vi "Query_Dust_Event_v2.vi"(8 "error in (no error)":errorcluster) -> (0 "error out":errorcluster)   [LabVIEW 2015]
uses:
  Controls/Constraints.ctl
  Controls/Graph.ctl
  Controls/Waveforms.ctl
  <vilib>/Utility/miscctls.llb/LVPointTypeDef.ctl
  <vilib>/addons/h5labview/H5F_mode.ctl
  <userlib>/_OpenG.lib/array/array.llb/Remove Duplicates from 1D Array (String)__ogtk.vi
  <userlib>/_OpenG.lib/array/array.llb/Empty 1D Array (Variant)__ogtk.vi
  <userlib>/_OpenG.lib/array/array.llb/Search 1D Array (String)__ogtk.vi
  <userlib>/_OpenG.lib/array/array.llb/Empty 1D Array (I32)__ogtk.vi
  <userlib>/_OpenG.lib/array/array.llb/Index 1D Array Elements (String)__ogtk.vi
  <userlib>/_OpenG.lib/array/array.llb/Search 1D Array (I32)__ogtk.vi
  <userlib>/_OpenG.lib/array/array.llb/Delete Elements from 1D Array (I32)__ogtk.vi
  <userlib>/_OpenG.lib/array/array.llb/Search 1D Array (Variant)__ogtk.vi
  <userlib>/_OpenG.lib/comparison/comparison.llb/Boolean Changed__ogtk.vi
  <vilib>/Utility/file.llb/Write To Spreadsheet File (string).vi
  <userlib>/_OpenG.lib/array/array.llb/Search 1D Array (U64)__ogtk.vi
  <userlib>/_OpenG.lib/array/array.llb/Sort 1D Array (U64)__ogtk.vi
  <userlib>/_OpenG.lib/array/array.llb/Delete Elements from 1D Array (U64)__ogtk.vi
  <vilib>/addons/h5labview/H5File.lvlib
panel:
  out "Updating...":bool
  out "Week":dbl
  out "Last Metadata Name":string
  in  "Tab Control":T1(tab)
  in  "Limit to":i64=10000 min=0 step=1000
  in  "Limit no. of\nplotted events":bool=TRUE
  in  "Experiment Group":string
  in  "Plot":bool
  in  "Select Names":bool
  in  "Save Plot Metadata":bool caption="Save Metadata"
  in  "Show Names":bool
  out "Plotted Metadata Slide":u8(slide) scale=0.0..100.0
  in  "Save Image":bool
  out "Plot Radius?":bool
  out "Constrained Distribution":T2
  in  "Experiment Name":string
  in  "Save Plot Waveforms":bool caption="Save Waveforms"
  out "Plotted Waveforms Slide":u8(slide) scale=0.0..100.0
  in  "Reset Constraints to Default":bool
  out "Number of Matching Events:":i32
  out "Description for Experiment Name:":string caption="Experiment Description:"
  out "Percentage of triggers that fit constraints:":dbl format="%#_4g%"
  out "Total Number of triggers:":i64
  in  "Constraints":T3={"Upper Timestamp Range"=timestamp(0 s since 1904-01-01), "Lower Timestamp Range"=timestamp(0 s since 1904-01-01), "Experiment Group:"="", "Experiment Name:"=[], "Upper Velocity Limit (km/s)"=299792.0, "Lower Velocity Limit (km/s)"=0.0, "Upper Mass Limit (kg)"=1.0, "Lower Mass Limit (kg)"=0.0, "name array"=[], "Estimate Quality"={0.0, 5.0}} {"Estimate Quality" scale=-5.0..5.0; "Lower Mass Limit (kg)" min=-1.0 max=1.0 step=1e-20; "Upper Mass Limit (kg)" min=-1.0 max=1.0 step=1e-20; "Lower Velocity Limit (km/s)" min=-1.0 max=299792000.0; "Upper Velocity Limit (km/s)" min=-1.0 max=299792000.0}
  out "Dust Type":string
  in  "Radius (µm)":dbl=2.0
  in  "Mass (kg)":dbl=2.638602750087072e-13 min=1e-20 max=1e-10
  in  "Velocity (km/s)":dbl=1.0 min=0.001 max=200.0
  out "Density (g/cc)":dbl
  in  "Reset Visible Time":bool caption="Save Metadata"
  out "Number of selected waveforms":i32=10
  in  "Select None":bool
  in  "Select All":bool
  in  "Selected?":bool
  in  "Limit waveforms to":i64=10
  in  "Plot Waveforms":bool
  in  "Show errored waveforms":bool
  in  "Set to plot constraints":bool
  out "Waveforms":T4[](array[typedef])
  in  "Waveform Select Names":bool
  in  "Waveforms Experiment Name":string
  in  "Waveform Show Names":bool
  in  "Waveforms Experiment Group":string
  in  "Waveform Constraints":T3 {"Estimate Quality" scale=0.0..5.0; "Lower Mass Limit (kg)" min=0.0 step=1e-20; "Upper Mass Limit (kg)" min=0.0 step=1e-20}
  out "Selected Waveforms":u64[](array[numeric])
  out "Selected Waveforms Slide":u8(slide) scale=0.0..100.0
  in  "Save Selected Waveforms":bool caption="Save Waveforms"
  out "Selected Metadata Slide":u8(slide) scale=0.0..100.0
  in  "Save Selected Metadata":bool caption="Save Metadata"
  in  "Time Visible":dbl=5000.0 min=0.0 step=1000.0
  out "Max Time":dbl=5000.0
  out "Multipliers":dbl[](array[numeric])
  in  "If this was the big acc...":bool
  in  "Sensitivity:":dbl=12100000000000.0
  in  "Vnoise Estimate:":dbl=0.005
  in  "Pelletron Voltage (MV):":dbl=2.17 caption="Needle Voltage (MV):"
  out "Test":bool caption="Test Database in use:"
  out "Test 2":bool caption="Production Database in use:"
  in  "Small?":bool
  in  "Clear Errors":bool
  in  "Exit":bool
  # "Query Dust Event V2"
  # "Go to Desktop/Accelerator/Documentation/SQL Column Translations.xlsx\nfor info about the Estimate Quality metric"
  # "events"
  # "Cursor"
  # "events"
  # "Plot Settings:"
  # "Error Status:"
  # "ODBC Connection Status:"
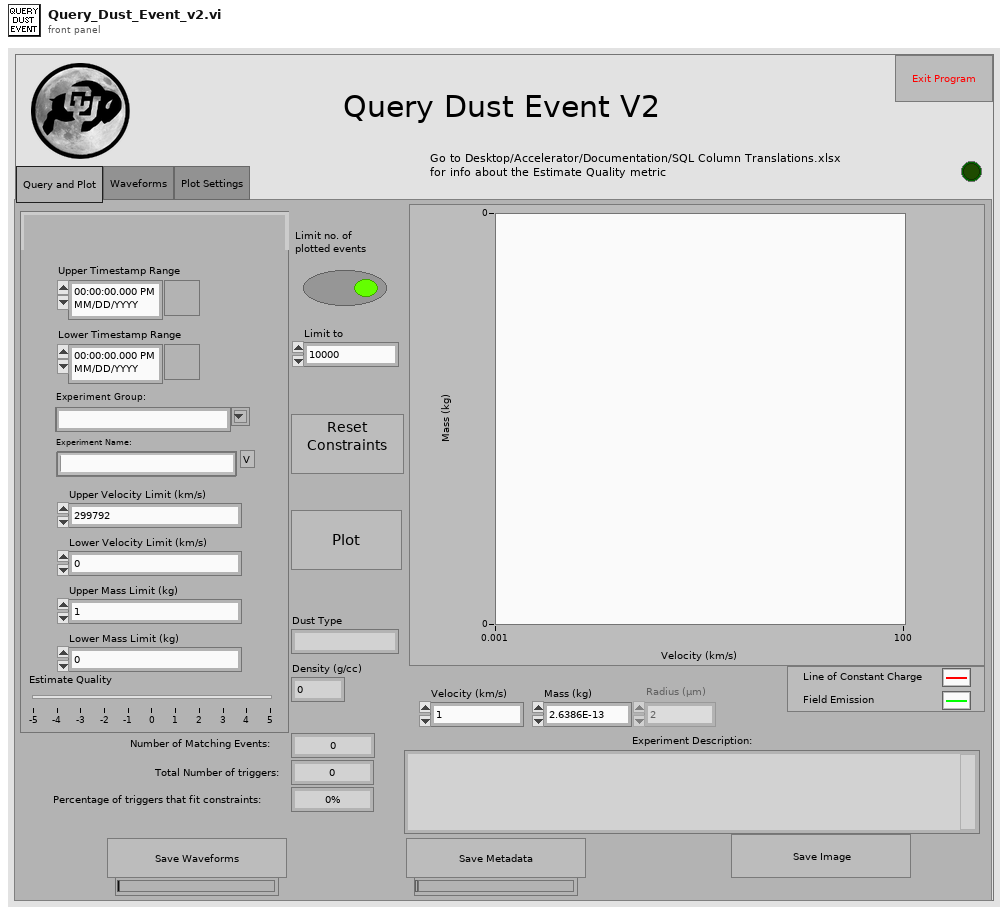
[diagram p1: front panel]
types:
  T1 = enum32{"Query and Plot", "Waveforms", "Plot Settings"}
  T2 = typedef "Graph.ctl" = cluster{cluster{"Vnoise":dbl, "Vnoise":dbl}[]}[]
  T3 = typedef "Constraints.ctl" = cluster{"Upper Timestamp Range":timestamp, "Lower Timestamp Range":timestamp, "Experiment Group:":string, "Experiment Name:":i32[], "Upper Velocity Limit (km/s)":dbl, "Lower Velocity Limit (km/s)":dbl, "Upper Mass Limit (kg)":dbl, "Lower Mass Limit (kg)":dbl, "name array":string[], "Estimate Quality":cluster{dbl, dbl}}
  T4 = typedef "Waveforms.ctl" = cluster{"id_dust_event":u64, "Time Stamp":timestamp, "Velocity":dbl, "Mass":dbl, "Charge":dbl, "Radius":dbl, "Waveform Graph":sgl[][], "Quality":i32}
  T5 = enum8{"Enabled", "Disabled", "Disabled and Grayed Out"}
  T6 = typedef "LVPointTypeDef.ctl" = cluster{"Horizontal":i16, "Vertical":i16}
  T7 = typedef "H5File.lvlib/H5F_mode.ctl" = enum16{"read-only", "read-write", "overwrite", "create new", "open or create"}
  T8 = typedef "Query_Dust_Event.ctl" = cluster{"Dust Event ID":i64, "Integer Timestamp":i64, "Velocity":dbl, "Mass":dbl, "Charge":sgl, "Radius":sgl, "Passed_3rd_Detector":i8, "High Voltage":sgl, "+ High Voltage Supply":sgl, "- High Voltage Supply":sgl, "HV Control Difference":sgl, "Vacuum Pressure":sgl, "Radiation":sgl, "Column Current":sgl, "Lost Charge":sgl, "Chain Current":sgl, "Control High Voltage":sgl, "Current Group Name:":string, "Current Experiment Name:":string, "Current Experiment Description:":string, "Estimate Source":T9, "Estimate Quality":i8, "File Location":T10, "Dust Type":string, "Dust Density":sgl}
  T9 = typedef "Estimate_source.ctl" = i8
  T10 = typedef "File_location.ctl" = i8
  T11 = cluster{"Upper Timestamp Range":timestamp, "Lower Timestamp Range":timestamp, "Experiment Group:":string, "Experiment Name:":i32[], "Upper Velocity Limit (km/s)":dbl, "Lower Velocity Limit (km/s)":dbl, "Upper Mass Limit (kg)":dbl, "Lower Mass Limit (kg)":dbl, "name array":string[], "Estimate Quality":cluster{dbl, dbl}}
  T12 = typedef "imagedata.ctl" = cluster{"image type":i32, "image depth":i32, "image":u8[], "mask":u8[], "colors":u32[], "Rectangle":cluster{"left":i16, "top":i16, "right":i16, "bottom":i16}}
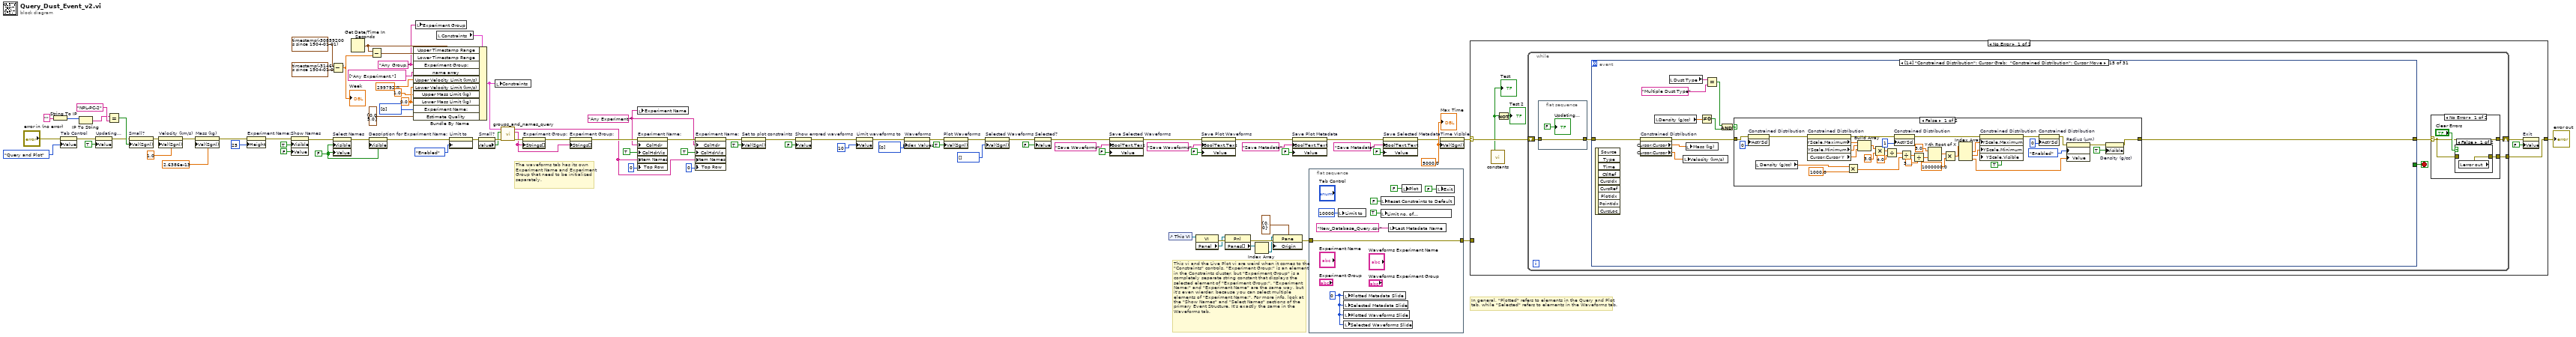
[diagram p0: block diagram]
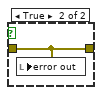
[diagram p2: hidden frame]
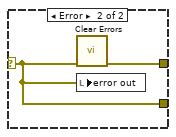
[diagram p3: hidden frame]
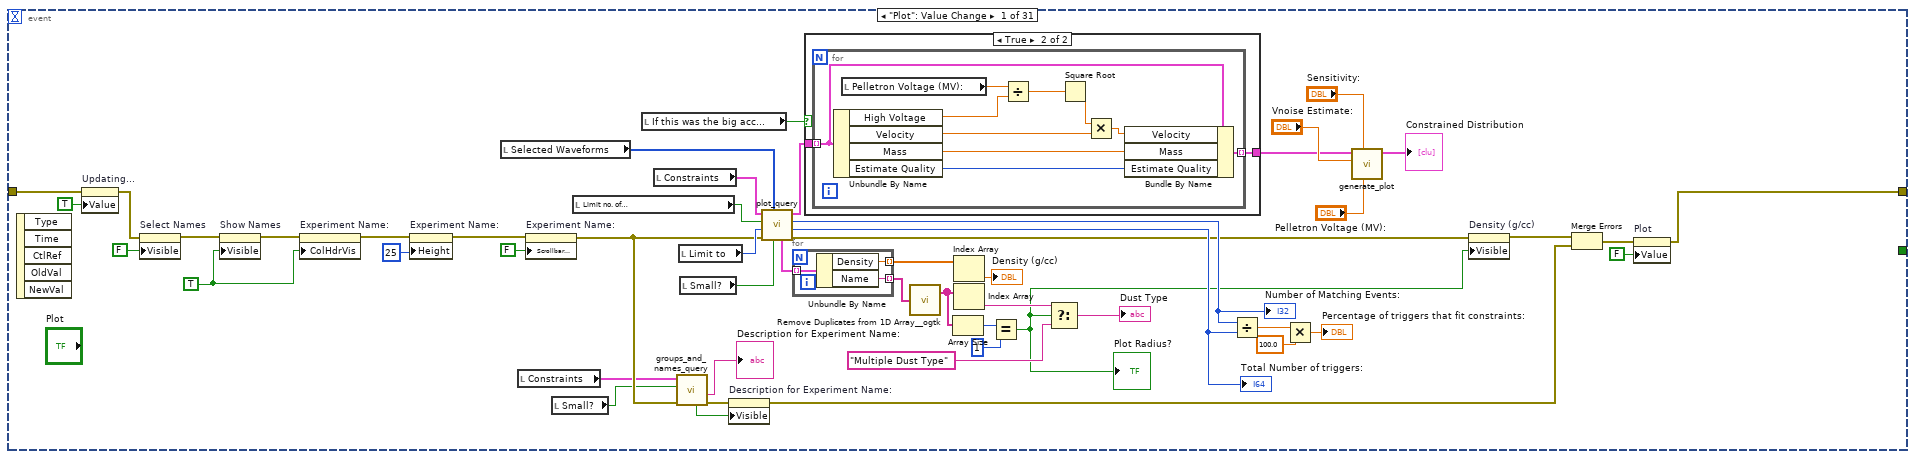
[diagram p4: hidden frame]
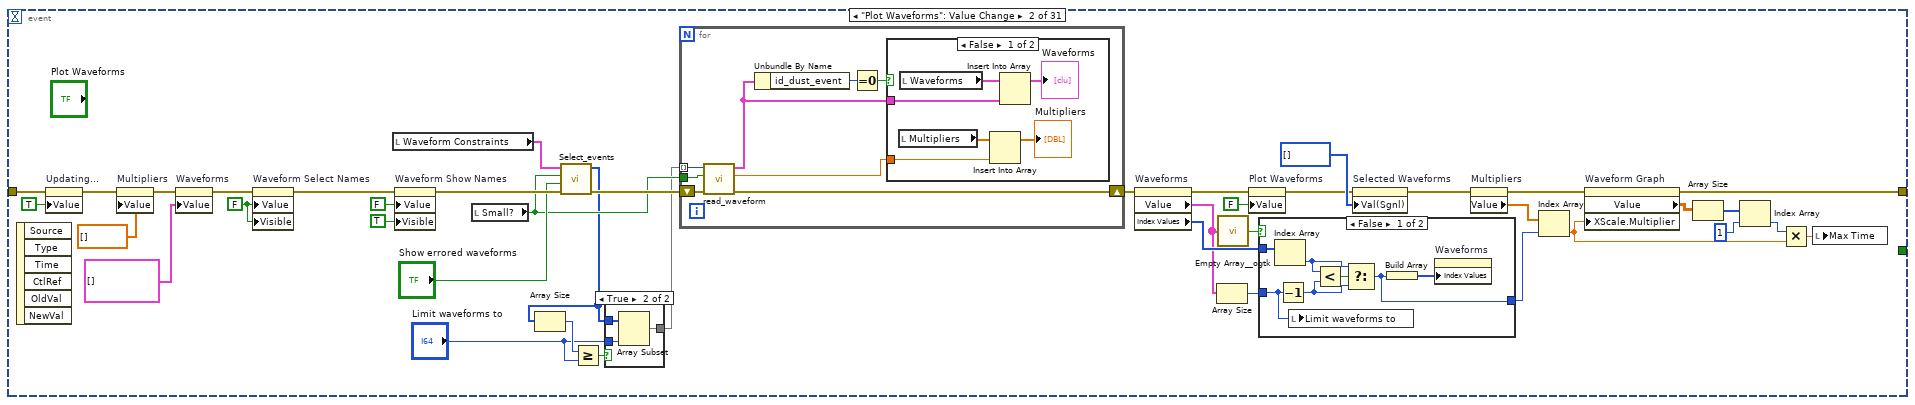
[diagram p6: hidden frame]
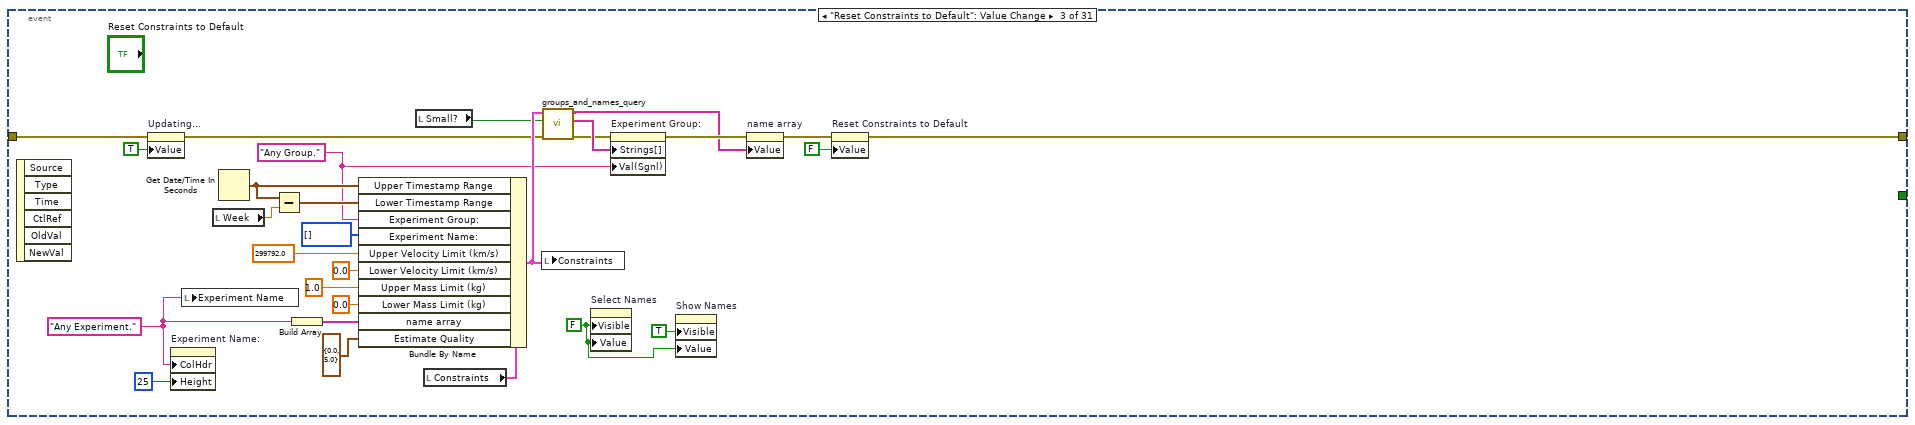
[diagram p10: hidden frame]
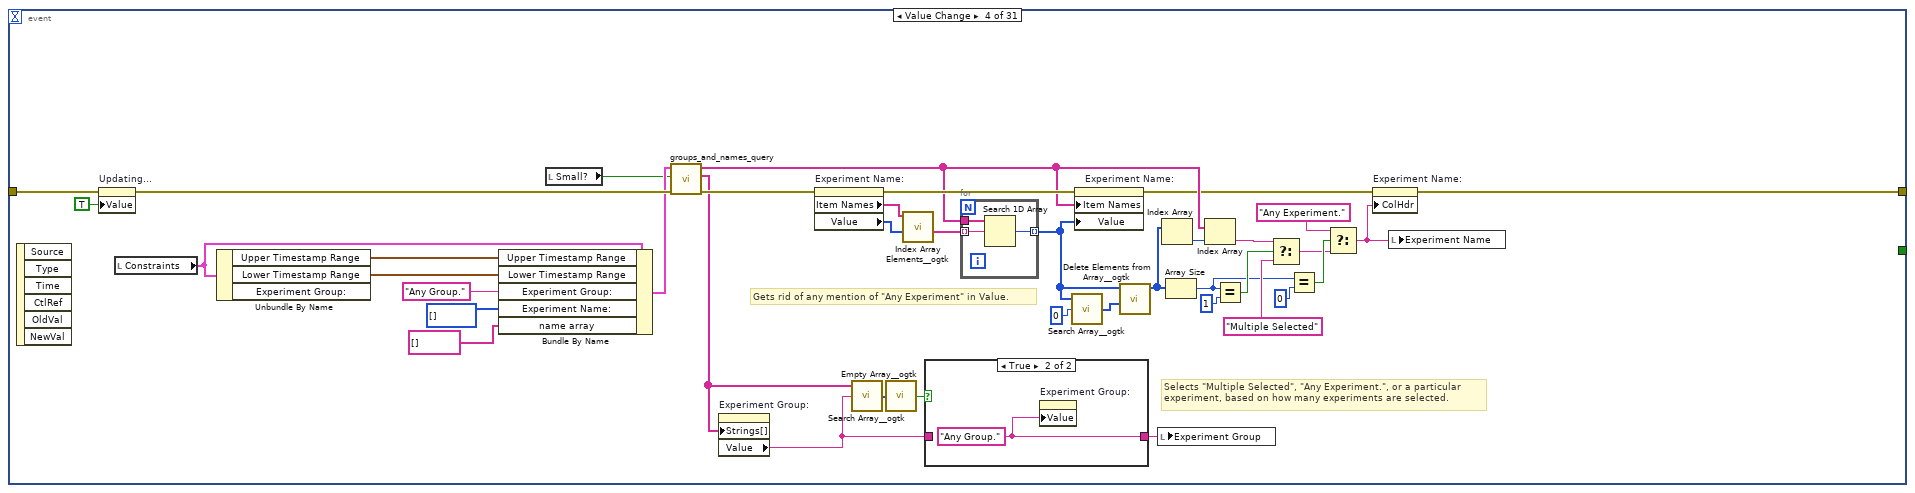
[diagram p11: hidden frame]
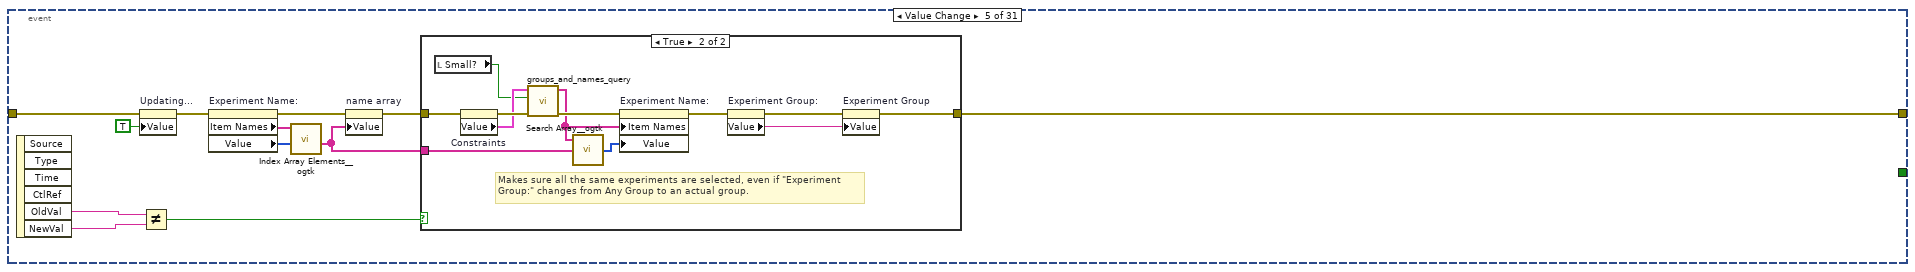
[diagram p13: hidden frame]
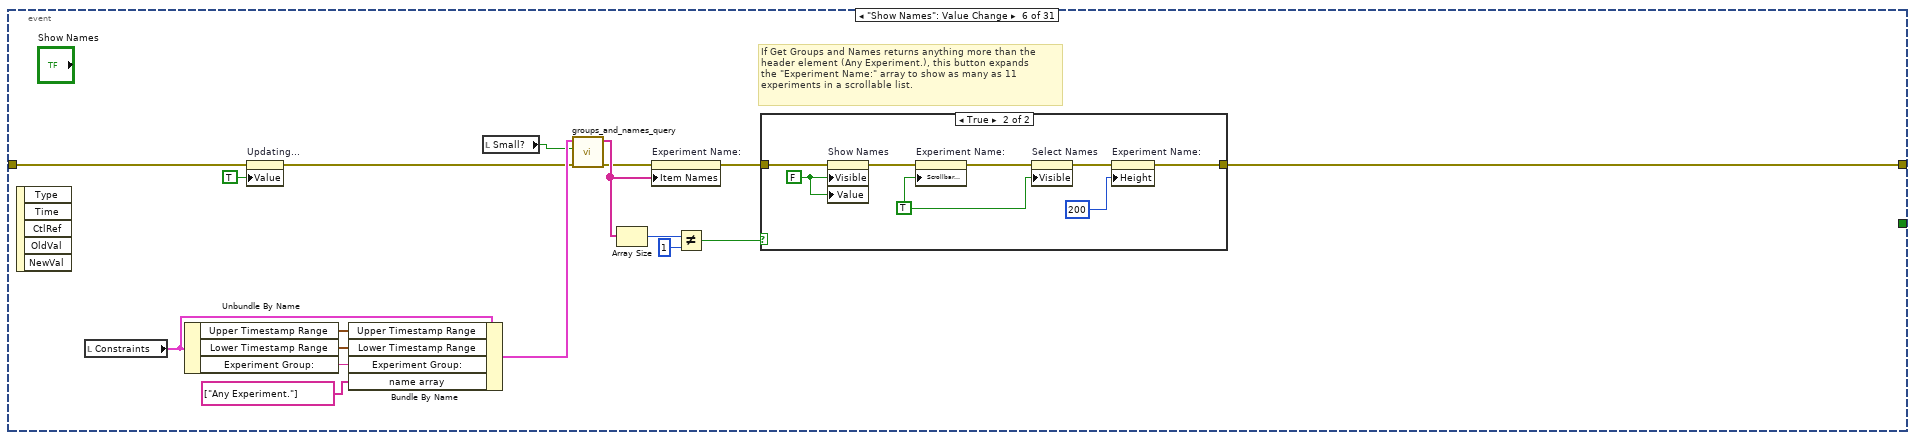
[diagram p15: hidden frame]
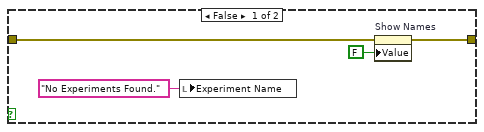
[diagram p16: hidden frame]
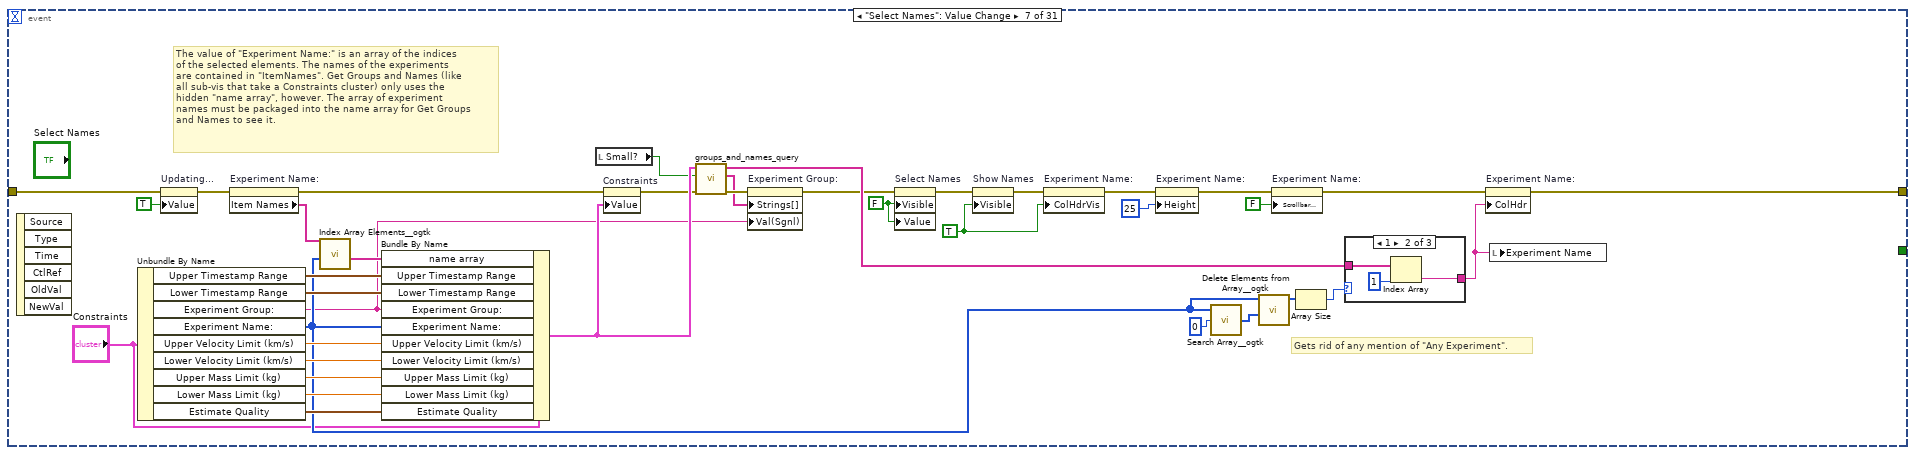
[diagram p17: hidden frame]
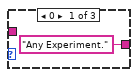
[diagram p18: hidden frame]
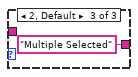
[diagram p19: hidden frame]
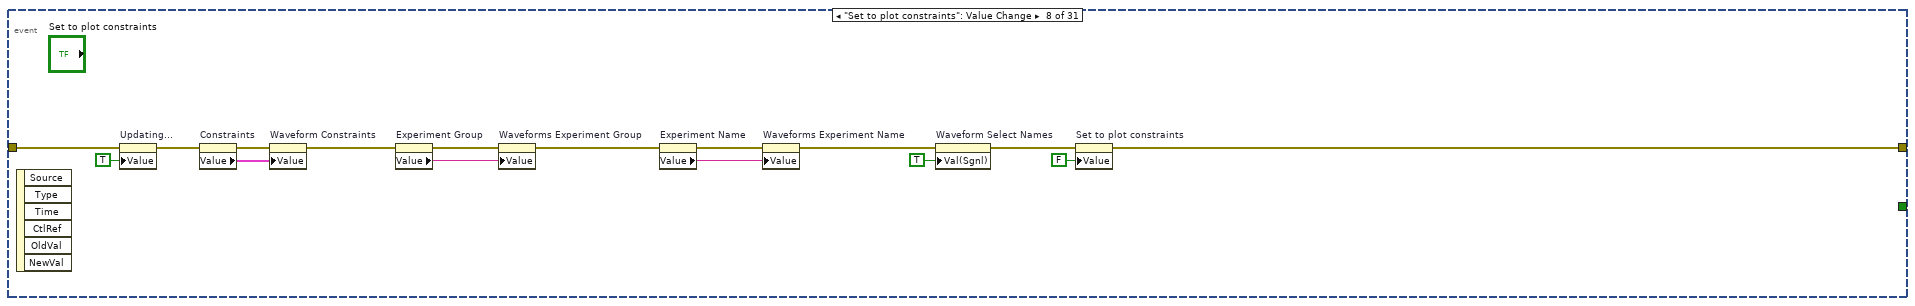
[diagram p20: hidden frame]
diagram:
  w4 = 5000.0 ("Min Time")
  w66 = 0.0 ("Lower Mass Limit (kg)")
  w63 = "Any Group." ("element")
  w71 = FALSE ("Visible")
  w28 = "Any Experiment." ("element")
  # "This vi and the Live Plot vi are weird when it comes to the\n\"Constraints\" controls. \"Experiment Group:\" is an element\nin the Constraints cluster, but \"Experiment Group\" is a\ncompletely separate string constant that displays the\nselected element of \"Experiment Group:\". \"Experiment\nName:\" and \"Experiment Name\" are the same way, but\nit's even wierder, because you can select multiple\nelements of \"Experiment Name:\". For more info, look at\nthe \"Show Names\" and \"Select Names\" sections of the\nprimary Event Structure. It's exactly the same in the\nWaveforms tab."
  # "In general, \"Plotted\" refers to elements in the Query and Plot\ntab, while \"Selected\" refers to elements in the Waveforms tab."
  # "The waveforms tab has its own\nExperiment Name and Experiment\nGroup that need to be initialized\nseparately."
  n1 = String To IP(1:"" ("name")) -> (0:w48:u32)
  n2 = property on="Tab Control" class="TabCtl (strict)"(error in="error in (no error)", "Value"=T1."Query and Plot" ("Tab Control")) -> (error out=w38:errorcluster)  [unwired: 1 in, 1 out]
  n3 = IP To String(2:w48) -> (0:w46:string)  [unwired: 1 in]
  n4 = property on="Updating..." class="Bool (strict)"(error in=w38, "Value"=TRUE ("Updating...")) -> (error out=w37:errorcluster)  [unwired: 1 in, 1 out]
  n5 = Equal?(x=w46, y="NPL-PC-2" ("x")) -> (x = y?=w60:bool)
  n6 = property on="Small?" class="Bool (strict)"(error in=w37, "Val(Sgnl)"=w60) -> (error out=w36:errorcluster)  [unwired: 1 in, 1 out]
  n7 = property on="Velocity (km/s)" class="DigNum (strict)"(error in=w36, "Val(Sgnl)"=1.0 ("Value (Signaling)")) -> (error out=w53:errorcluster)  [unwired: 1 in, 1 out]
  n8 = property on="Mass (kg)" class="DigNum (strict)"(error in=w53, "Val(Sgnl)"=2.6386e-13 ("Value (Signaling)")) -> (error out=w50:errorcluster)  [unwired: 1 in, 1 out]
  n9 = property on="Experiment Name:" class="LstBox (strict)"(error in=w50, "Height"=25 ("x")) -> (error out=w69:errorcluster)  [unwired: 1 in, 1 out]
  n10 = property on="Show Names" class="Bool (strict)"(error in=w69, "Visible"=TRUE, "Value"=FALSE ("Show Names")) -> (error out=w86:errorcluster)  [unwired: 1 in, 1 out]
  n11 = Subtract(x=timestamp(-30859200 s since 1904-01-01) ("current time"), y=timestamp(-31464000 s since 1904-01-01) ("current time")) -> (x-y=w68:dbl)
  "Week" <- w68
  n12 = property on="Select Names" class="Bool (strict)"(error in=w86, "Visible"=w71, "Value"=w71) -> (error out=w85:errorcluster)  [unwired: 1 in, 1 out]
  n13 = Get Date/Time In Seconds() -> (seconds since 1Jan1904=w88:timestamp)
  n14 = property on="Description for Experiment Name:" class="Str"(error in=w85, "Visible"=w71) -> (error out=w56:errorcluster)  [unwired: 1 in, 1 out]
  n15 = Subtract(x=w88, y=w68) -> (x-y=w87:timestamp)
  n16 = local write "Experiment Group"(w63) -> ()
  n17 = local read "Constraints"() -> (w91:T3)
  n18 = Bundle By Name(cluster=w91, "Upper Timestamp Range"=w88, "Lower Timestamp Range"=w87, "Experiment Group:"=w63, "name array"=string[] ["Any Experiment."] ("Experiment Name:"), "Upper Velocity Limit (km/s)"=299792.0, "Lower Velocity Limit (km/s)"=w66, "Upper Mass Limit (kg)"=1.0 ("Lower Mass Limit (kg)"), "Lower Mass Limit (kg)"=w66, "Experiment Name:"=i32[] [0], "Estimate Quality"=cluster{dbl, dbl} {0.0, 5.0} ("Dust Quality")) -> (w82:T3)
  n19 = property on="Limit to" class="DigNum (strict)"(error in=w56, "DisabledEnum"=T5."Enabled" ("Disabled")) -> (error out=w54:errorcluster)  [unwired: 1 in, 1 out]
  n20 = property on="Small?" class="Bool (strict)"(error in=w54) -> (error out=w59:errorcluster, "Value"=w58:bool)  [unwired: 1 in, 1 out]
  n21 = local write "Constraints"(w82) -> ()
  n22 = call "groups_and_names_query.vi"("error in (no error)"=w59, "Small?"=w58, "Constraints"=w82) -> ("error out"=w62:errorcluster, "Groups"=w26:string[], "Names"=w27:string[])  [unwired: 4 in, 2 out]
  n23 = property on="Experiment Group:" class="CmbBox"(error in=w62, "Strings[]"=w26) -> (error out=w33:errorcluster)  [unwired: 1 in, 1 out]
  n24 = property on="Experiment Group:" class="CmbBox"(error in=w33, "Strings[]"=w26) -> (error out=w32:errorcluster)  [unwired: 1 in, 1 out]
  n25 = local write "Experiment Name"(w28) -> ()
  n26 = property on="Experiment Name:" class="LstBox (strict)"(error in=w32, "ColHdr"=w28, "ColHdrVis"=TRUE ("Visible Items:Column Header Visible"), "Item Names"=w27, "Top Row"=0) -> (error out=w29:errorcluster)  [unwired: 1 in, 1 out]
  n27 = property on="Experiment Name:" class="LstBox (strict)"(error in=w29, "ColHdr"=w28, "ColHdrVis"=TRUE ("Visible Items:Column Header Visible"), "Item Names"=w27, "Top Row"=0) -> (error out=w18:errorcluster)  [unwired: 1 in, 1 out]
  n28 = property on="Set to plot constraints" class="Bool (strict)"(error in=w18, "Val(Sgnl)"=TRUE ("Value (Signaling)")) -> (error out=w39:errorcluster)  [unwired: 1 in, 1 out]
  n29 = property on="Show errored waveforms" class="Bool (strict)"(error in=w39, "Value"=FALSE ("Show errored waveforms")) -> (error out=w40:errorcluster)  [unwired: 1 in, 1 out]
  n30 = property on="Limit waveforms to" class="DigNum (strict)"(error in=w40, "Value"=u64 10 ("Limit waveforms to")) -> (error out=w35:errorcluster)  [unwired: 1 in, 1 out]
  n31 = property on="Waveforms" class="Arr (strict)"(error in=w35, "Index Values"=u32[] [0]) -> (error out=w25:errorcluster)  [unwired: 1 in, 1 out]
  n32 = property on="Plot Waveforms" class="Bool (strict)"(error in=w25, "Val(Sgnl)"=TRUE ("Value (Signaling)")) -> (error out=w22:errorcluster)  [unwired: 1 in, 1 out]
  n33 = property on="Selected Waveforms" class="Arr (strict)"(error in=w22, "Val(Sgnl)"=u64[] [] ("Selected Waveforms")) -> (error out=w20:errorcluster)  [unwired: 1 in, 1 out]
  n34 = property on="Selected?" class="Bool (strict)"(error in=w20, "Value"=FALSE ("Selected?")) -> (error out=w14:errorcluster)  [unwired: 1 in, 1 out]
  n35 = property on="Save Selected Waveforms" class="Bool (strict)"(error in=w14, "BoolText.Text"="Save Waveforms" ("f"), "Value"=FALSE ("Save Selected Waveforms")) -> (error out=w11:errorcluster)  [unwired: 1 in, 1 out]
  n36 = control-ref of="This VI"() -> (w79:refnum<vi>)
  n37 = property class="VI"(reference=w79) -> (error out=w78:errorcluster, "Panel"=w77:refnum<vi>)  [unwired: 1 in, 1 out]
  n38 = property on="Save Plot Waveforms" class="Bool (strict)"(error in=w11, "BoolText.Text"="Save Waveforms" ("f"), "Value"=FALSE ("Save Selected Waveforms")) -> (error out=w6:errorcluster)  [unwired: 1 in, 1 out]
  n39 = property class="Pnl"(reference=w77, error in=w78) -> (error out=w76:errorcluster, "Panes[]"=w75:refnum<vi>[])  [unwired: 1 out]
  n40 = Index Array(array=w75) -> (element=w74:refnum<vi>)  [unwired: 1 in]
  n41 = property class="Pane"(reference=w74, error in=w76, "Origin"=T6 {"Horizontal"=0, "Vertical"=0}) -> (error out=w23:errorcluster)  [unwired: 1 out]
  n42 = property on="Save Plot Metadata" class="Bool (strict)"(error in=w6, "BoolText.Text"="Save Metadata" ("f"), "Value"=FALSE ("Save Selected Waveforms")) -> (error out=w5:errorcluster)  [unwired: 1 in, 1 out]
  n43 = flat-sequence {
    tunnel: w23 -> [w93]
    tunnel: [w93] -> w17
    frame #0 {
      w92 = u8 0 ("Plotted Metadata Slide")
      n44 = local write "Limit to"(i64 10000 ("Limit to")) -> ()
      n45 = local write "Plotted Metadata Slide"(w92) -> ()
      n46 = local write "Selected Metadata Slide"(w92) -> ()
      n47 = local write "Plotted Waveforms Slide"(w92) -> ()
      n48 = local write "Selected Waveforms Slide"(w92) -> ()
      n49 = local write "Reset Constraints to Default"(FALSE) -> ()
      n50 = local write "Limit no. of\nplotted events"(TRUE ("write metadata only")) -> ()
      n51 = local write "Last Metadata Name"("New_Database_Query.csv") -> ()
      n52 = local write "Plot"(FALSE) -> ()
      n53 = local write "Exit"(FALSE) -> ()
    }
  }
  n54 = property on="Save Selected Metadata" class="Bool (strict)"(error in=w5, "BoolText.Text"="Save Metadata" ("f"), "Value"=FALSE ("Save Selected Waveforms")) -> (error out=w2:errorcluster)  [unwired: 1 in, 1 out]
  n55 = property on="Time Visible" class="DigNum (strict)"(error in=w2, "Val(Sgnl)"=w4) -> (error out=w3:errorcluster)  [unwired: 1 in, 1 out]
  n56 = case shown="No Error" w3 {
    selector: w3 -> [w101 w1072]
    tunnel: w17 -> [_ _]
    tunnel: [w102 w1072] -> w1
    frame No Error {
      n57 = call "constants.vi"() -> ("Testing"=w100:bool)  [unwired: 3 out]
      "Test" <- w100
      n58 = Not(x=w100) -> (.not. x?=→"Test 2":bool)
      n59 = while {
        shift-right: [w107] -> w104
        shift-left: w101 -> [w111]
        tunnel: [w106] -> w102
        stop <- w109 stop-if-true
        n60 = flat-sequence {
          tunnel: [w119] -> w110
          tunnel: w111 -> [w119]
          frame #0 {
            "Updating..." <- FALSE ("Updating...")
          }
        }
        n61 = event shown="[14] \"Constrained Distribution\": Cursor Grab;  \"Constrained Distribution\": Cursor Move" {
          selector: _ -> [_ _ _ _ _ _ _ _ _ _ _ _ _ _ _ _ _ _ _ _ _ _ _ _ _ _ _ _ _ _ _]
          dyn-events: _ -> [_ _ _ _ _ _ _ _ _ _ _ _ _ _ _ _ _ _ _ _ _ _ _ _ _ _ _ _ _ _ _]
          timeout: _ -> [_ _ _ _ _ _ _ _ _ _ _ _ _ _ _ _ _ _ _ _ _ _ _ _ _ _ _ _ _ _ _]
          tunnel: w110 -> [w141 w223 w266 w319 w336 w355 w396 w423 w476 w493 w513 w554 w587 w616 w647 w700 w717 w739 w761 w825 w877 w898 w917 w926 w949 w967 w974 w980 w983 w1027 w1070]
          tunnel: [w136 w199 w256 w292 w332 w367 w389 w427 w439 w483 w508 w539 w577 w593 w646 w699 w721 w734 w741 w807 w870 w889 w918 w923 w938 w960 w971 w976 w985 w1030 w1070] -> w108
          tunnel: [_ _ _ _ _ _ _ _ _ _ _ _ _ _ _ _ _ _ _ _ _ _ _ _ _ _ _ _ _ _ "Exit"] -> w109
          event "Plot": Value Change {
            w170 = TRUE ("Visible")
            n62 = event-data() -> ()  [unwired: 1 in, 5 out]
            n63 = property on="Updating..." class="Bool (strict)"(error in=w141, "Value"=TRUE ("Updating...")) -> (error out=w140:errorcluster)  [unwired: 1 in, 1 out]
            n64 = property on="Select Names" class="Bool (strict)"(error in=w140, "Visible"=FALSE) -> (error out=w167:errorcluster)  [unwired: 1 in, 1 out]
            n65 = property on="Show Names" class="Bool (strict)"(error in=w167, "Visible"=w170) -> (error out=w166:errorcluster)  [unwired: 1 in, 1 out]
            n66 = property on="Experiment Name:" class="LstBox (strict)"(error in=w166, "ColHdrVis"=w170) -> (error out=w157:errorcluster)  [unwired: 1 in, 1 out]
            n67 = property on="Experiment Name:" class="LstBox (strict)"(error in=w157, "Height"=u32 25 ("Size:Height")) -> (error out=w165:errorcluster)  [unwired: 1 in, 1 out]
            n68 = local read "Selected Waveforms"() -> (w124:u64[])
            n69 = local read "Constraints"() -> (w133:T3)
            n70 = property on="Experiment Name:" class="LstBox (strict)"(error in=w165, "Scrollbar Visible"=FALSE ("Visible Items:Vertical Scrollbar Visible")) -> (error out=w137:errorcluster)  [unwired: 1 in, 1 out]
            n71 = local read "Small?"() -> (w129:bool)
            n72 = local read "Limit no. of\nplotted events"() -> (w144:bool)
            n73 = local read "If this was the big acc..."() -> (w126:bool)
            n74 = local read "Constraints"() -> (w146:T3)
            n75 = call "groups_and_names_query.vi"("error in (no error)"=w137, "Small?"=w129, "Constraints"=w133) -> ("error out"=w123:errorcluster, "Description"=→"Description for Experiment Name:":string, "Description Returned?"=w145:bool)  [unwired: 4 in, 2 out]
            n76 = local read "Limit to"() -> (w143:i64)
            n77 = local read "Small?"() -> (w130:bool)
            n78 = property on="Description for Experiment Name:" class="Str"(error in=w123, "Visible"=w145) -> (error out=w122:errorcluster)  [unwired: 1 in, 1 out]
            n79 = call "plot_query.vi"("Small?"=w130, "Selected Dust Events"=w124, "error in (no error)"=w137, "Limit no. of events"=w143, "Limited?"=w144, "Constraints"=w146) -> ("error out"=w121:errorcluster, "Total Number of triggers"=w139:u64, "Number of Matching Events"=w138:u64, "Dust Array"=w128:T8[], "Dust Info"=w151:cluster{"Density":dbl, "Name":string}[])  [unwired: 1 in]
            "Number of Matching Events:" <- w138
            "Total Number of triggers:" <- w139
            n80 = for {
              tunnel: [w187] -> w148 mode=indexing
              tunnel: [w186] -> w156 mode=indexing
              tunnel: w151 -> [w185] mode=indexing
              n81 = Unbundle By Name(w185) -> ("Density"=w187:dbl, "Name"=w186:string)
            }
            n82 = case shown="True" w126 {
              tunnel: w128 -> [w172 w174]
              tunnel: [w172 w173] -> w127
              frame False {
              }
              frame True {
                n83 = for {
                  tunnel: w174 -> [w184] mode=indexing
                  tunnel: [w183] -> w173 mode=indexing
                  n84 = Unbundle By Name(w184) -> ("High Voltage"=w179:sgl, "Velocity"=w178:dbl, "Mass"=w181:dbl, "Estimate Quality"=w182:i8)
                  n85 = local read "Pelletron Voltage (MV):"() -> (w180:dbl)
                  n86 = Divide(x=w180, y=w179) -> (x/y=w176:dbl)
                  n87 = Square Root(x=w176) -> (sqrt(x)=w175:dbl)
                  n88 = Multiply(x=w175, y=w178) -> (x*y=w177:dbl)
                  n89 = Bundle By Name(cluster=w184, "Velocity"=w177, "Mass"=w181, "Estimate Quality"=w182) -> (w183:T8)
                }
              }
            }
            n90 = call-poly <userlib>:"Remove Duplicates from 1D Array__ogtk.vi"("Input Array"=w156) -> ("Output Array"=w149:string[])  [unwired: 1 out]
            n91 = Array Size(array=w149) -> (size(s)=w155:i32)
            n92 = Index Array(array=w148) -> (element=→"Density (g/cc)":dbl)  [unwired: 1 in]
            n93 = Index Array(array=w149) -> (element=w152:string)  [unwired: 1 in]
            n94 = Equal?(x=w155, y=1) -> (x = y?=w131:bool)
            "Plot Radius?" <- w131
            n95 = Select(t=w152, s=w131, f="Multiple Dust Type" ("t")) -> (s? t:f=→"Dust Type":string)
            n96 = Divide(x=w138, y=w139) -> (x/y=w162:dbl)
            n97 = Multiply(x=w162, y=100.0) -> (x*y=→"Percentage of triggers that fit constraints:":dbl)
            n98 = call "generate_plot.vi"("High Voltage"="Pelletron Voltage (MV):", "Sens"="Sensitivity:", "Vnoise"="Vnoise Estimate:", "Dust Array"=w127) -> ("Dust Distribution"=→"Constrained Distribution":T2)  [unwired: 7 in]
            n99 = property on="Density (g/cc)" class="DigNum (strict)"(error in=w121, "Visible"=w131) -> (error out=w132:errorcluster)  [unwired: 1 in, 1 out]
            n100 = Merge Errors(w132, w122) -> (w135:errorcluster)
            n101 = property on="Plot" class="Bool (strict)"(error in=w135, "Value"=FALSE ("Plot")) -> (error out=w136:errorcluster)  [unwired: 1 in, 1 out]
          }
          event "Plot Waveforms": Value Change {
            w227 = FALSE ("Waveform Select Names")
            n102 = event-data() -> ()  [unwired: 1 in, 6 out]
            n103 = property on="Updating..." class="Bool (strict)"(error in=w223, "Value"=TRUE ("Updating...")) -> (error out=w189:errorcluster)  [unwired: 1 in, 1 out]
            n104 = property on="Multipliers" class="Arr (strict)"(error in=w189, "Value"=dbl[] [] ("Multipliers")) -> (error out=w190:errorcluster)  [unwired: 1 in, 1 out]
            n105 = property on="Waveforms" class="Arr (strict)"(error in=w190, "Value"=T4[] [] ("Waveforms")) -> (error out=w220:errorcluster)  [unwired: 1 in, 1 out]
            n106 = property on="Waveform Select Names" class="Bool (strict)"(error in=w220, "Value"=w227, "Visible"=w227) -> (error out=w228:errorcluster)  [unwired: 1 in, 1 out]
            n107 = local read "Waveform Constraints"() -> (w221:T3)
            n108 = property on="Waveform Show Names" class="Bool (strict)"(error in=w228, "Value"=FALSE ("Waveform Select Names"), "Visible"=TRUE) -> (error out=w222:errorcluster)  [unwired: 1 in, 1 out]
            n109 = local read "Small?"() -> (w216:bool)
            n110 = call "Select_events.vi"("error in (no error)"=w222, "Select errored events"="Show errored waveforms", "Small?"=w216, "Constraints"=w221) -> ("error out"=w217:errorcluster, "Dust Events"=w204:i64[])  [unwired: 6 in]
            n111 = Array Size(array=w204) -> (size(s)=w205:i32)
            n112 = Greater Or Equal?(x=w205, y="Limit waveforms to") -> (x >= y?=w206:bool)
            n113 = case shown="True" w206 {
              tunnel: w204 -> [w229 w232]
              tunnel: "Limit waveforms to" -> [_ w231]
              tunnel: [w229 w230] -> w212
              frame False {
              }
              frame True {
                n114 = Array Subset(array=w232, length=w231) -> (w230:i64[])  [unwired: 1 in]
              }
            }
            n115 = for {
              tunnel: w212 -> [w247] mode=indexing
              shift-right: [w241] -> w215
              shift-left: w217 -> [w246]
              tunnel: w216 -> [w245]
              n116 = call "read_waveform.vi"("error in (no error)"=w246, "Small?"=w245, "Dust Event ID"=w247) -> ("error out"=w241:errorcluster, "multiplier"=w240:dbl, "Waveform"=w244:T4)  [unwired: 6 in]
              n117 = Unbundle By Name(w244) -> ("id_dust_event"=w243:u64)
              n118 = Equal To 0?(x=w243) -> (x = 0?=w242:bool)
              n119 = case shown="False" w242 {
                tunnel: w244 -> [w251 _]
                tunnel: w240 -> [w248 _]
                frame False {
                  n120 = local read "Multipliers"() -> (w249:dbl[])
                  n121 = local read "Waveforms"() -> (w252:T4[])
                  n122 = Insert Into Array(array=w249, new element=w248) -> (→"Multipliers":dbl[])  [unwired: 1 in]
                  n123 = Insert Into Array(array=w252, new element=w251) -> (→"Waveforms":T4[])  [unwired: 1 in]
                }
                frame True {
                }
              }
            }
            n124 = property on="Waveforms" class="Arr (strict)"(error in=w215) -> (error out=w210:errorcluster, "Value"=w207:T4[], "Index Values"=w214:u32[])  [unwired: 1 in, 1 out]
            n125 = Array Size(array=w207) -> (size(s)=w208:i32)
            n126 = call-poly <userlib>:"Empty Array__ogtk.vi"("Array"=w207) -> ("Empty Array?"=w213:bool)  [unwired: 8 in]
            n127 = property on="Plot Waveforms" class="Bool (strict)"(error in=w210, "Value"=FALSE ("Value (Signaling)")) -> (error out=w202:errorcluster)  [unwired: 1 in, 1 out]
            n128 = case shown="False" w213 {
              tunnel: w214 -> [w239 _]
              tunnel: w208 -> [w234 _]
              tunnel: [w233 _] -> w197
              frame False {
                n129 = Index Array(array=w239) -> (element=w237:u32)  [unwired: 1 in]
                n130 = Decrement(x=w234) -> (x-1=w236:i32)
                n131 = local write "Limit waveforms to"(w234) -> ()
                n132 = Less?(x=w237, y=w236) -> (x < y?=w238:bool)
                n133 = Select(t=w237, s=w238, f=w236) -> (s? t:f=w233:u32)
                n134 = Build Array(w233) -> (w235:u32[])
                n135 = property on="Waveforms" class="Arr (strict)"("Index Values"=w235) -> ()  [unwired: 2 in, 2 out]
              }
              frame True {
              }
            }
            n136 = property on="Selected Waveforms" class="Arr (strict)"(error in=w202, "Val(Sgnl)"=u64[] [] ("Value (Signaling)")) -> (error out=w201:errorcluster)  [unwired: 1 in, 1 out]
            n137 = property on="Multipliers" class="Arr (strict)"(error in=w201) -> (error out=w200:errorcluster, "Value"=w198:dbl[])  [unwired: 1 in, 1 out]
            n138 = Index Array(array=w198, index=w197) -> (element=w192:dbl)
            n139 = property on="Waveform Graph" class="WFGraph (strict)"(error in=w200, "XScale.Multiplier"=w192) -> (error out=w199:errorcluster, "Value"=w193:sgl[][])  [unwired: 1 in, 1 out]
            n140 = Array Size(array=w193) -> (size(s)=w194:i32[])
            n141 = Index Array(array=w194, index=1) -> (element=w196:i32)
            n142 = Multiply(x=w196, y=w192) -> (x*y=w191:dbl)
            n143 = local write "Max Time"(w191) -> ()
          }
          event "Reset Constraints to Default": Value Change {
            w254 = "Any Group." ("Experiment Group")
            w277 = FALSE ("Visible")
            w271 = "Any Experiment." ("element")
            n144 = event-data() -> ()  [unwired: 1 in, 6 out]
            n145 = property on="Updating..." class="Bool (strict)"(error in=w266, "Value"=TRUE ("Updating...")) -> (error out=w265:errorcluster)  [unwired: 1 in, 1 out]
            n146 = property on="Experiment Name:" class="LstBox (strict)"("ColHdr"=w271, "Height"=u32 25 ("Size:Height")) -> ()  [unwired: 2 in, 2 out]
            n147 = local write "Experiment Name"(w271) -> ()
            n148 = local read "Week"() -> (w255:dbl)
            n149 = Get Date/Time In Seconds() -> (seconds since 1Jan1904=w276:timestamp)
            n150 = Subtract(x=w276, y=w255) -> (x-y=w275:timestamp)
            n151 = Build Array(w271) -> (w270:string[])
            n152 = local read "Small?"() -> (w264:bool)
            n153 = local read "Constraints"() -> (w273:T3)
            n154 = Bundle By Name(cluster=w273, "Upper Timestamp Range"=w276, "Lower Timestamp Range"=w275, "Experiment Group:"=w254, "Experiment Name:"=i32[] [], "Upper Velocity Limit (km/s)"=299792.0, "Lower Velocity Limit (km/s)"=0.0, "Upper Mass Limit (kg)"=1.0, "Lower Mass Limit (kg)"=0.0, "name array"=w270, "Estimate Quality"=cluster{dbl, dbl} {0.0, 5.0}) -> (w268:T3)
            n155 = local write "Constraints"(w268) -> ()
            n156 = call "groups_and_names_query.vi"("error in (no error)"=w265, "Small?"=w264, "Constraints"=w268) -> ("error out"=w280:errorcluster, "Groups"=w281:string[], "Names"=w274:string[])  [unwired: 4 in, 2 out]
            n157 = property on="Select Names" class="Bool (strict)"("Visible"=w277, "Value"=w277) -> ()  [unwired: 2 in, 2 out]
            n158 = property on="Experiment Group:" class="CmbBox"(error in=w280, "Strings[]"=w281, "Val(Sgnl)"=w254) -> (error out=w279:errorcluster)  [unwired: 1 in, 1 out]
            n159 = property on="Show Names" class="Bool (strict)"("Visible"=TRUE, "Value"=w277) -> ()  [unwired: 2 in, 2 out]
            n160 = property on="name array" class="Arr (strict)"(error in=w279, "Value"=w274) -> (error out=w257:errorcluster)  [unwired: 1 in, 1 out]
            n161 = property on="Reset Constraints to Default" class="Bool (strict)"(error in=w257, "Value"=FALSE ("Reset Constraints to Default")) -> (error out=w256:errorcluster)  [unwired: 1 in, 1 out]
          }
          event Value Change {
            # "Selects \"Multiple Selected\", \"Any Experiment.\", or a particular\nexperiment, based on how many experiments are selected."
            # "Gets rid of any mention of \"Any Experiment\" in Value."
            n162 = event-data() -> ()  [unwired: 1 in, 6 out]
            n163 = property on="Updating..." class="Bool (strict)"(error in=w319, "Value"=TRUE ("Updating...")) -> (error out=w313:errorcluster)  [unwired: 1 in, 1 out]
            n164 = local read "Constraints"() -> (w287:T3)
            n165 = Unbundle By Name(w287) -> ("Upper Timestamp Range"=w316:timestamp, "Lower Timestamp Range"=w315:timestamp)  [unwired: 1 out]
            n166 = Bundle By Name(cluster=w287, "Upper Timestamp Range"=w316, "Lower Timestamp Range"=w315, "Experiment Group:"="Any Group.", "Experiment Name:"=i32[] [], "name array"=string[] []) -> (w312:T3)
            n167 = local read "Small?"() -> (w290:bool)
            n168 = call "groups_and_names_query.vi"("error in (no error)"=w313, "Small?"=w290, "Constraints"=w312) -> ("error out"=w311:errorcluster, "Groups"=w291:string[], "Names"=w294:string[])  [unwired: 4 in, 2 out]
            n169 = property on="Experiment Group:" class="CmbBox"("Strings[]"=w291) -> ("Value"=w285:string)  [unwired: 2 in, 2 out]
            n170 = property on="Experiment Name:" class="LstBox (strict)"(error in=w311) -> (error out=w307:errorcluster, "Item Names"=w310:string[], "Value"=w309:i32[])  [unwired: 1 in, 1 out]
            n171 = call-poly <userlib>:"Search Array__ogtk.vi"("Array"=w291, "Element Data"=w285) -> ("Indices of Elements"=w289:i32[])  [unwired: 7 in]
            n172 = call-poly <userlib>:"Empty Array__ogtk.vi"("Array"=w289) -> ("Empty Array?"=w288:bool)  [unwired: 8 in]
            n173 = call-poly <userlib>:"Index Array Elements__ogtk.vi"("indices"=w309, "array"=w310) -> ("elements"=w308:string[])  [unwired: 9 in]
            n174 = case shown="True" w288 {
              tunnel: [w324 w325] -> w286
              tunnel: w285 -> [w324 _]
              frame False {
              }
              frame True {
                w325 = "Any Group." ("Experiment Group")
                n175 = property on="Experiment Group:" class="CmbBox"("Value"=w325) -> ()  [unwired: 2 in, 2 out]
              }
            }
            n176 = for {
              tunnel: w308 -> [w323] mode=indexing
              tunnel: [w322] -> w284 mode=indexing
              tunnel: w294 -> [w321]
              n177 = Search 1D Array(1D array=w321, element=w323) -> (index of element=w322:i32)  [unwired: 1 in]
            }
            n178 = call-poly <userlib>:"Search Array__ogtk.vi"("Array"=w284, "Element Data"=0) -> ("Indices of Elements"=w300:i32[])  [unwired: 7 in]
            n179 = property on="Experiment Name:" class="LstBox (strict)"(error in=w307, "Item Names"=w294, "Value"=w284) -> (error out=w293:errorcluster)  [unwired: 1 in, 1 out]
            n180 = call-poly <userlib>:"Delete Elements from Array__ogtk.vi"("indices"=w300, "array"=w284) -> ("array w/ subset deleted"=w283:i32[])  [unwired: 8 in, 1 out]
            n181 = local write "Experiment Group"(w286) -> ()
            n182 = Index Array(array=w283) -> (element=w282:i32)  [unwired: 1 in]
            n183 = Array Size(array=w283) -> (size(s)=w298:i32)
            n184 = Index Array(array=w294, index=w282) -> (element=w302:string)
            n185 = Equal?(x=w298, y=1) -> (x = y?=w304:bool)
            n186 = Select(t=w302, s=w304, f="Multiple Selected") -> (s? t:f=w295:string)
            n187 = Equal?(x=w298, y=0) -> (x = y?=w296:bool)
            n188 = Select(t="Any Experiment.", s=w296, f=w295) -> (s? t:f=w306:string)
            n189 = property on="Experiment Name:" class="LstBox (strict)"(error in=w293, "ColHdr"=w306) -> (error out=w292:errorcluster)  [unwired: 1 in, 1 out]
            n190 = local write "Experiment Name"(w306) -> ()
          }
          event Value Change {
            n191 = event-data() -> ("OldVal"=w334:string, "NewVal"=w335:string)  [unwired: 1 in, 4 out]
            n192 = property on="Updating..." class="Bool (strict)"(error in=w336, "Value"=TRUE ("Updating...")) -> (error out=w329:errorcluster)  [unwired: 1 in, 1 out]
            n193 = Not Equal?(x=w334, y=w335) -> (x != y?=w333:bool)
            n194 = property on="Experiment Name:" class="LstBox (strict)"(error in=w329) -> (error out=w328:errorcluster, "Item Names"=w331:string[], "Value"=w330:i32[])  [unwired: 1 in, 1 out]
            n195 = call-poly <userlib>:"Index Array Elements__ogtk.vi"("indices"=w330, "array"=w331) -> ("elements"=w326:string[])  [unwired: 9 in]
            n196 = property on="name array" class="Arr (strict)"(error in=w328, "Value"=w326) -> (error out=w327:errorcluster)  [unwired: 1 in, 1 out]
            n197 = case shown="True" w333 {
              tunnel: w327 -> [w338 w343]
              tunnel: [w338 w344] -> w332
              tunnel: w326 -> [_ w342]
              frame False {
              }
              frame True {
                # "Makes sure all the same experiments are selected, even if \"Experiment\nGroup:\" changes from Any Group to an actual group."
                n198 = local read "Small?"() -> (w341:bool)
                n199 = property on="Constraints" class="Clust (strict)"(error in=w343) -> (error out=w350:errorcluster, "Value"=w349:T11)  [unwired: 1 in, 1 out]
                n200 = call "groups_and_names_query.vi"("error in (no error)"=w350, "Small?"=w341, "Constraints"=w349) -> ("error out"=w348:errorcluster, "Names"=w346:string[])  [unwired: 4 in, 3 out]
                n201 = call-poly <userlib>:"Search Array__ogtk.vi"("Array"=w346, "Element Data"=w342) -> ("Indices of Elements"=w347:i32[])  [unwired: 7 in]
                n202 = property on="Experiment Name:" class="LstBox (strict)"(error in=w348, "Item Names"=w346, "Value"=w347) -> (error out=w345:errorcluster)  [unwired: 1 in, 1 out]
                n203 = property on="Experiment Group:" class="CmbBox"(error in=w345) -> (error out=w340:errorcluster, "Value"=w339:string)  [unwired: 1 in, 1 out]
                n204 = property on="Experiment Group" class="Str"(error in=w340, "Value"=w339) -> (error out=w344:errorcluster)  [unwired: 1 in, 1 out]
              }
            }
          }
          event "Show Names": Value Change {
            # "If Get Groups and Names returns anything more than the\nheader element (Any Experiment.), this button expands\nthe \"Experiment Name:\" array to show as many as 11\nexperiments in a scrollable list."
            n205 = event-data() -> ()  [unwired: 1 in, 5 out]
            n206 = local read "Constraints"() -> (w361:T3)
            n207 = Unbundle By Name(w361) -> ("Upper Timestamp Range"=w358:timestamp, "Lower Timestamp Range"=w359:timestamp, "Experiment Group:"=w360:string)
            n208 = property on="Updating..." class="Bool (strict)"(error in=w355, "Value"=TRUE ("Updating...")) -> (error out=w354:errorcluster)  [unwired: 1 in, 1 out]
            n209 = Bundle By Name(cluster=w361, "Upper Timestamp Range"=w358, "Lower Timestamp Range"=w359, "Experiment Group:"=w360, "name array"=string[] ["Any Experiment."]) -> (w362:T3)
            n210 = local read "Small?"() -> (w351:bool)
            n211 = call "groups_and_names_query.vi"("error in (no error)"=w354, "Small?"=w351, "Constraints"=w362) -> ("error out"=w363:errorcluster, "Names"=w364:string[])  [unwired: 4 in, 3 out]
            n212 = Array Size(array=w364) -> (size(s)=w365:i32)
            n213 = property on="Experiment Name:" class="LstBox (strict)"(error in=w363, "Item Names"=w364) -> (error out=w353:errorcluster)  [unwired: 1 in, 1 out]
            n214 = Not Equal?(x=w365, y=1) -> (x != y?=w352:bool)
            n215 = case shown="True" w352 {
              tunnel: [w370 w379] -> w367
              tunnel: w353 -> [w368 w378]
              frame False {
                n216 = local write "Experiment Name"("No Experiments Found." ("Experiment Name")) -> ()
                n217 = property on="Show Names" class="Bool (strict)"(error in=w368, "Value"=FALSE ("Show Names")) -> (error out=w370:errorcluster)  [unwired: 1 in, 1 out]
              }
              frame True {
                w372 = FALSE ("Visible")
                w376 = TRUE ("Visible Items:Vertical Scrollbar Visible")
                n218 = property on="Show Names" class="Bool (strict)"(error in=w378, "Visible"=w372, "Value"=w372) -> (error out=w375:errorcluster)  [unwired: 1 in, 1 out]
                n219 = property on="Experiment Name:" class="LstBox (strict)"(error in=w375, "Scrollbar Visible"=w376) -> (error out=w374:errorcluster)  [unwired: 1 in, 1 out]
                n220 = property on="Select Names" class="Bool (strict)"(error in=w374, "Visible"=w376) -> (error out=w377:errorcluster)  [unwired: 1 in, 1 out]
                n221 = property on="Experiment Name:" class="LstBox (strict)"(error in=w377, "Height"=200 ("x")) -> (error out=w379:errorcluster)  [unwired: 1 in, 1 out]
              }
            }
          }
          event "Select Names": Value Change {
            w403 = TRUE ("Visible")
            w401 = FALSE ("Visible")
            # "The value of \"Experiment Name:\" is an array of the indices\nof the selected elements. The names of the experiments\nare contained in \"ItemNames\". Get Groups and Names (like\nall sub-vis that take a Constraints cluster) only uses the\nhidden \"name array\", however. The array of experiment\nnames must be packaged into the name array for Get Groups\nand Names to see it."
            # "Gets rid of any mention of \"Any Experiment\"."
            n222 = event-data() -> ()  [unwired: 1 in, 6 out]
            n223 = Unbundle By Name("Constraints") -> ("Upper Timestamp Range"=w417:timestamp, "Lower Timestamp Range"=w416:timestamp, "Experiment Group:"=w384:string, "Experiment Name:"=w392:i32[], "Upper Velocity Limit (km/s)"=w415:dbl, "Lower Velocity Limit (km/s)"=w414:dbl, "Upper Mass Limit (kg)"=w413:dbl, "Lower Mass Limit (kg)"=w412:dbl, "Estimate Quality"=w410:cluster{dbl, dbl})
            n224 = property on="Updating..." class="Bool (strict)"(error in=w396, "Value"=TRUE ("Updating...")) -> (error out=w405:errorcluster)  [unwired: 1 in, 1 out]
            n225 = property on="Experiment Name:" class="LstBox (strict)"(error in=w405) -> (error out=w393:errorcluster, "Item Names"=w395:string[])  [unwired: 1 in, 1 out]
            n226 = call-poly <userlib>:"Index Array Elements__ogtk.vi"("indices"=w392, "array"=w395) -> ("elements"=w394:string[])  [unwired: 9 in]
            n227 = Bundle By Name(cluster="Constraints", "name array"=w394, "Upper Timestamp Range"=w417, "Lower Timestamp Range"=w416, "Experiment Group:"=w384, "Experiment Name:"=w392, "Upper Velocity Limit (km/s)"=w415, "Lower Velocity Limit (km/s)"=w414, "Upper Mass Limit (kg)"=w413, "Lower Mass Limit (kg)"=w412, "Estimate Quality"=w410) -> (w409:T3)
            n228 = local read "Small?"() -> (w385:bool)
            n229 = property on="Constraints" class="Clust (strict)"(error in=w393, "Value"=w409) -> (error out=w408:errorcluster)  [unwired: 1 in, 1 out]
            n230 = call "groups_and_names_query.vi"("error in (no error)"=w408, "Small?"=w385, "Constraints"=w409) -> ("error out"=w411:errorcluster, "Groups"=w407:string[], "Names"=w390:string[])  [unwired: 4 in, 2 out]
            n231 = property on="Experiment Group:" class="CmbBox"(error in=w411, "Strings[]"=w407, "Val(Sgnl)"=w384) -> (error out=w383:errorcluster)  [unwired: 1 in, 1 out]
            n232 = property on="Select Names" class="Bool (strict)"(error in=w383, "Visible"=w401, "Value"=w401) -> (error out=w404:errorcluster)  [unwired: 1 in, 1 out]
            n233 = property on="Show Names" class="Bool (strict)"(error in=w404, "Visible"=w403) -> (error out=w402:errorcluster)  [unwired: 1 in, 1 out]
            n234 = property on="Experiment Name:" class="LstBox (strict)"(error in=w402, "ColHdrVis"=w403) -> (error out=w391:errorcluster)  [unwired: 1 in, 1 out]
            n235 = property on="Experiment Name:" class="LstBox (strict)"(error in=w391, "Height"=u32 25 ("Size:Height")) -> (error out=w397:errorcluster)  [unwired: 1 in, 1 out]
            n236 = call-poly <userlib>:"Search Array__ogtk.vi"("Array"=w392, "Element Data"=0) -> ("Indices of Elements"=w388:i32[])  [unwired: 7 in]
            n237 = call-poly <userlib>:"Delete Elements from Array__ogtk.vi"("indices"=w388, "array"=w392) -> ("array w/ subset deleted"=w387:i32[])  [unwired: 8 in, 1 out]
            n238 = property on="Experiment Name:" class="LstBox (strict)"(error in=w397, "Scrollbar Visible"=FALSE ("Visible Items:Vertical Scrollbar Visible")) -> (error out=w399:errorcluster)  [unwired: 1 in, 1 out]
            n239 = Array Size(array=w387) -> (size(s)=w381:i32)
            n240 = case shown="1" w381 {
              tunnel: w390 -> [_ w421 _]
              tunnel: ["Any Experiment." ("t") w419 "Multiple Selected" ("f")] -> w380
              frame 0 {
              }
              frame 1 {
                n241 = Index Array(array=w421, index=1) -> (element=w419:string)
              }
              frame 2, Default {
              }
            }
            n242 = property on="Experiment Name:" class="LstBox (strict)"(error in=w399, "ColHdr"=w380) -> (error out=w389:errorcluster)  [unwired: 1 in, 1 out]
            n243 = local write "Experiment Name"(w380) -> ()
          }
          event "Set to plot constraints": Value Change {
            n244 = event-data() -> ()  [unwired: 1 in, 6 out]
            n245 = property on="Updating..." class="Bool (strict)"(error in=w423, "Value"=TRUE ("Updating...")) -> (error out=w424:errorcluster)  [unwired: 1 in, 1 out]
            n246 = property on="Constraints" class="Clust (strict)"(error in=w424) -> (error out=w438:errorcluster, "Value"=w437:T11)  [unwired: 1 in, 1 out]
            n247 = property on="Waveform Constraints" class="Clust (strict)"(error in=w438, "Value"=w437) -> (error out=w434:errorcluster)  [unwired: 1 in, 1 out]
            n248 = property on="Experiment Group" class="Str"(error in=w434) -> (error out=w435:errorcluster, "Value"=w436:string)  [unwired: 1 in, 1 out]
            n249 = property on="Waveforms Experiment Group" class="Str"(error in=w435, "Value"=w436) -> (error out=w431:errorcluster)  [unwired: 1 in, 1 out]
            n250 = property on="Experiment Name" class="Str"(error in=w431) -> (error out=w433:errorcluster, "Value"=w432:string)  [unwired: 1 in, 1 out]
            n251 = property on="Waveforms Experiment Name" class="Str"(error in=w433, "Value"=w432) -> (error out=w430:errorcluster)  [unwired: 1 in, 1 out]
            n252 = property on="Waveform Select Names" class="Bool (strict)"(error in=w430, "Val(Sgnl)"=TRUE ("Waveform Select Names")) -> (error out=w426:errorcluster)  [unwired: 1 in, 1 out]
            n253 = property on="Set to plot constraints" class="Bool (strict)"(error in=w426, "Value"=FALSE ("Set to plot constraints")) -> (error out=w427:errorcluster)  [unwired: 1 in, 1 out]
          }
          event Value Change {
            # "Selects \"Multiple Selected\", \"Any Experiment.\", or a particular\nexperiment, based on how many experiments are selected."
            # "Gets rid of any mention of \"Any Experiment\" in Value."
            n254 = event-data() -> ()  [unwired: 1 in, 6 out]
            n255 = local read "Waveform Constraints"() -> (w445:T3)
            n256 = property on="Updating..." class="Bool (strict)"(error in=w476, "Value"=TRUE ("Updating...")) -> (error out=w470:errorcluster)  [unwired: 1 in, 1 out]
            n257 = Unbundle By Name(w445) -> ("Upper Timestamp Range"=w473:timestamp, "Lower Timestamp Range"=w472:timestamp)  [unwired: 1 out]
            n258 = Bundle By Name(cluster=w445, "Upper Timestamp Range"=w473, "Lower Timestamp Range"=w472, "Experiment Group:"="Any Group.", "Experiment Name:"=i32[] [], "name array"=string[] []) -> (w469:T3)
            n259 = local read "Small?"() -> (w448:bool)
            n260 = call "groups_and_names_query.vi"("error in (no error)"=w470, "Small?"=w448, "Constraints"=w469) -> ("error out"=w468:errorcluster, "Groups"=w449:string[], "Names"=w451:string[])  [unwired: 4 in, 2 out]
            n261 = property on="Experiment Group:" class="CmbBox"("Strings[]"=w449) -> ("Value"=w443:string)  [unwired: 2 in, 2 out]
            n262 = property on="Experiment Name:" class="LstBox (strict)"(error in=w468) -> (error out=w464:errorcluster, "Item Names"=w467:string[], "Value"=w466:i32[])  [unwired: 1 in, 1 out]
            n263 = call-poly <userlib>:"Search Array__ogtk.vi"("Array"=w449, "Element Data"=w443) -> ("Indices of Elements"=w447:i32[])  [unwired: 7 in]
            n264 = call-poly <userlib>:"Empty Array__ogtk.vi"("Array"=w447) -> ("Empty Array?"=w446:bool)  [unwired: 8 in]
            n265 = call-poly <userlib>:"Index Array Elements__ogtk.vi"("indices"=w466, "array"=w467) -> ("elements"=w465:string[])  [unwired: 9 in]
            n266 = case shown="True" w446 {
              tunnel: [w481 w482] -> w444
              tunnel: w443 -> [w481 _]
              frame False {
              }
              frame True {
                w482 = "Any Group." ("Experiment Group")
                n267 = property on="Experiment Group:" class="CmbBox"("Value"=w482) -> ()  [unwired: 2 in, 2 out]
              }
            }
            n268 = for {
              tunnel: w465 -> [w480] mode=indexing
              tunnel: [w479] -> w442 mode=indexing
              tunnel: w451 -> [w478]
              n269 = Search 1D Array(1D array=w478, element=w480) -> (index of element=w479:i32)  [unwired: 1 in]
            }
            n270 = call-poly <userlib>:"Search Array__ogtk.vi"("Array"=w442, "Element Data"=0) -> ("Indices of Elements"=w457:i32[])  [unwired: 7 in]
            n271 = property on="Experiment Name:" class="LstBox (strict)"(error in=w464, "Item Names"=w451, "Value"=w442) -> (error out=w450:errorcluster)  [unwired: 1 in, 1 out]
            n272 = call-poly <userlib>:"Delete Elements from Array__ogtk.vi"("indices"=w457, "array"=w442) -> ("array w/ subset deleted"=w441:i32[])  [unwired: 8 in, 1 out]
            n273 = local write "Waveforms Experiment Group"(w444) -> ()
            n274 = Index Array(array=w441) -> (element=w440:i32)  [unwired: 1 in]
            n275 = Array Size(array=w441) -> (size(s)=w455:i32)
            n276 = Index Array(array=w451, index=w440) -> (element=w459:string)
            n277 = Equal?(x=w455, y=1) -> (x = y?=w461:bool)
            n278 = Select(t=w459, s=w461, f="Multiple Selected") -> (s? t:f=w452:string)
            n279 = Equal?(x=w455, y=0) -> (x = y?=w453:bool)
            n280 = Select(t="Any Experiment.", s=w453, f=w452) -> (s? t:f=w463:string)
            n281 = property on="Experiment Name:" class="LstBox (strict)"(error in=w450, "ColHdr"=w463) -> (error out=w439:errorcluster)  [unwired: 1 in, 1 out]
            n282 = local write "Waveforms Experiment Name"(w463) -> ()
          }
          event Value Change {
            n283 = event-data() -> ("OldVal"=w491:string, "NewVal"=w492:string)  [unwired: 1 in, 4 out]
            n284 = property on="Updating..." class="Bool (strict)"(error in=w493, "Value"=TRUE ("Updating...")) -> (error out=w487:errorcluster)  [unwired: 1 in, 1 out]
            n285 = Not Equal?(x=w491, y=w492) -> (x != y?=w490:bool)
            n286 = property on="Experiment Name:" class="LstBox (strict)"(error in=w487) -> (error out=w486:errorcluster, "Item Names"=w489:string[], "Value"=w488:i32[])  [unwired: 1 in, 1 out]
            n287 = call-poly <userlib>:"Index Array Elements__ogtk.vi"("indices"=w488, "array"=w489) -> ("elements"=w484:string[])  [unwired: 9 in]
            n288 = property on="name array" class="Arr (strict)"(error in=w486, "Value"=w484) -> (error out=w485:errorcluster)  [unwired: 1 in, 1 out]
            n289 = case shown="True" w490 {
              tunnel: w485 -> [w495 w500]
              tunnel: [w495 w501] -> w483
              tunnel: w484 -> [_ w499]
              frame False {
              }
              frame True {
                n290 = property on="Waveform Constraints" class="Clust (strict)"(error in=w500) -> (error out=w507:errorcluster, "Value"=w506:T11)  [unwired: 1 in, 1 out]
                n291 = local read "Small?"() -> (w498:bool)
                n292 = call "groups_and_names_query.vi"("error in (no error)"=w507, "Small?"=w498, "Constraints"=w506) -> ("error out"=w505:errorcluster, "Names"=w503:string[])  [unwired: 4 in, 3 out]
                n293 = call-poly <userlib>:"Search Array__ogtk.vi"("Array"=w503, "Element Data"=w499) -> ("Indices of Elements"=w504:i32[])  [unwired: 7 in]
                n294 = property on="Experiment Name:" class="LstBox (strict)"(error in=w505, "Item Names"=w503, "Value"=w504) -> (error out=w502:errorcluster)  [unwired: 1 in, 1 out]
                n295 = property on="Experiment Group:" class="CmbBox"(error in=w502) -> (error out=w497:errorcluster, "Value"=w496:string)  [unwired: 1 in, 1 out]
                n296 = property on="Waveforms Experiment Group" class="Str"(error in=w497, "Value"=w496) -> (error out=w501:errorcluster)  [unwired: 1 in, 1 out]
              }
            }
          }
          event "Waveform Show Names": Value Change {
            n297 = event-data() -> ()  [unwired: 1 in, 5 out]
            n298 = local read "Waveform Constraints"() -> (w519:T3)
            n299 = Unbundle By Name(w519) -> ("Upper Timestamp Range"=w516:timestamp, "Lower Timestamp Range"=w517:timestamp, "Experiment Group:"=w518:string)
            n300 = property on="Updating..." class="Bool (strict)"(error in=w513, "Value"=TRUE ("Updating...")) -> (error out=w512:errorcluster)  [unwired: 1 in, 1 out]
            n301 = Bundle By Name(cluster=w519, "Upper Timestamp Range"=w516, "Lower Timestamp Range"=w517, "Experiment Group:"=w518, "name array"=string[] ["Any Experiment."]) -> (w520:T3)
            n302 = local read "Small?"() -> (w509:bool)
            n303 = call "groups_and_names_query.vi"("error in (no error)"=w512, "Small?"=w509, "Constraints"=w520) -> ("error out"=w521:errorcluster, "Names"=w522:string[])  [unwired: 4 in, 3 out]
            n304 = Array Size(array=w522) -> (size(s)=w523:i32)
            n305 = property on="Experiment Name:" class="LstBox (strict)"(error in=w521, "Item Names"=w522) -> (error out=w511:errorcluster)  [unwired: 1 in, 1 out]
            n306 = Not Equal?(x=w523, y=1) -> (x != y?=w510:bool)
            n307 = case shown="True" w510 {
              tunnel: [w527 w530] -> w508
              tunnel: w511 -> [w525 w535]
              frame False {
                n308 = property on="Waveform Show Names" class="Bool (strict)"(error in=w525, "Value"=FALSE ("Show Names")) -> (error out=w527:errorcluster)  [unwired: 1 in, 1 out]
                n309 = local write "Experiment Name"("No Experiments Found." ("Experiment Name")) -> ()
              }
              frame True {
                w531 = FALSE ("Visible")
                w534 = TRUE ("Visible Items:Vertical Scrollbar Visible")
                n310 = property on="Waveform Show Names" class="Bool (strict)"(error in=w535, "Visible"=w531, "Value"=w531) -> (error out=w533:errorcluster)  [unwired: 1 in, 1 out]
                n311 = property on="Experiment Name:" class="LstBox (strict)"(error in=w533, "Scrollbar Visible"=w534, "Height"=200 ("x")) -> (error out=w532:errorcluster)  [unwired: 1 in, 1 out]
                n312 = property on="Waveform Select Names" class="Bool (strict)"(error in=w532, "Visible"=w534) -> (error out=w530:errorcluster)  [unwired: 1 in, 1 out]
              }
            }
          }
          event "Waveform Select Names": Value Change {
            w555 = FALSE ("Visible")
            # "Gets rid of any mention of \"Any Experiment\" in Value."
            n313 = event-data() -> ()  [unwired: 1 in, 6 out]
            n314 = Unbundle By Name("Waveform Constraints") -> ("Upper Timestamp Range"=w571:timestamp, "Lower Timestamp Range"=w570:timestamp, "Experiment Group:"=w545:string, "Experiment Name:"=w550:i32[], "Upper Velocity Limit (km/s)"=w569:dbl, "Lower Velocity Limit (km/s)"=w568:dbl, "Upper Mass Limit (kg)"=w567:dbl, "Lower Mass Limit (kg)"=w566:dbl, "Estimate Quality"=w564:cluster{dbl, dbl})
            n315 = property on="Updating..." class="Bool (strict)"(error in=w554, "Value"=TRUE ("Updating...")) -> (error out=w559:errorcluster)  [unwired: 1 in, 1 out]
            n316 = property on="Experiment Name:" class="LstBox (strict)"(error in=w559) -> (error out=w551:errorcluster, "Item Names"=w553:string[])  [unwired: 1 in, 1 out]
            n317 = call-poly <userlib>:"Index Array Elements__ogtk.vi"("indices"=w550, "array"=w553) -> ("elements"=w552:string[])  [unwired: 9 in]
            n318 = Bundle By Name(cluster="Waveform Constraints", "name array"=w552, "Upper Timestamp Range"=w571, "Lower Timestamp Range"=w570, "Experiment Group:"=w545, "Experiment Name:"=w550, "Upper Velocity Limit (km/s)"=w569, "Lower Velocity Limit (km/s)"=w568, "Upper Mass Limit (kg)"=w567, "Lower Mass Limit (kg)"=w566, "Estimate Quality"=w564) -> (w563:T3)
            n319 = property on="Waveform Constraints" class="Clust (strict)"(error in=w551, "Value"=w563) -> (error out=w562:errorcluster)  [unwired: 1 in, 1 out]
            n320 = local read "Small?"() -> (w546:bool)
            n321 = call "groups_and_names_query.vi"("error in (no error)"=w562, "Small?"=w546, "Constraints"=w563) -> ("error out"=w565:errorcluster, "Groups"=w561:string[], "Names"=w538:string[])  [unwired: 4 in, 2 out]
            n322 = property on="Experiment Group:" class="CmbBox"(error in=w565, "Strings[]"=w561, "Val(Sgnl)"=w545) -> (error out=w544:errorcluster)  [unwired: 1 in, 1 out]
            n323 = call-poly <userlib>:"Search Array__ogtk.vi"("Array"=w550, "Element Data"=0) -> ("Indices of Elements"=w549:i32[])  [unwired: 7 in]
            n324 = call-poly <userlib>:"Delete Elements from Array__ogtk.vi"("indices"=w549, "array"=w550) -> ("array w/ subset deleted"=w548:i32[])  [unwired: 8 in, 1 out]
            n325 = Array Size(array=w548) -> (size(s)=w537:i32)
            n326 = property on="Waveform Select Names" class="Bool (strict)"(error in=w544, "Visible"=w555, "Value"=w555) -> (error out=w558:errorcluster)  [unwired: 1 in, 1 out]
            n327 = case shown="0" w537 {
              tunnel: ["Any Experiment." ("t") w573 "Multiple Selected" ("f")] -> w536
              tunnel: w538 -> [_ w574 _]
              frame 0 {
              }
              frame 1 {
                n328 = Index Array(array=w574, index=1) -> (element=w573:string)
              }
              frame 2, Default {
              }
            }
            n329 = property on="Waveform Show Names" class="Bool (strict)"(error in=w558, "Visible"=TRUE) -> (error out=w556:errorcluster)  [unwired: 1 in, 1 out]
            n330 = local write "Waveforms Experiment Name"(w536) -> ()
            n331 = property on="Experiment Name:" class="LstBox (strict)"(error in=w556, "ColHdrVis"=TRUE ("Visible Items:Column Header Visible"), "Height"=u32 25 ("Size:Height"), "Scrollbar Visible"=FALSE ("Visible Items:Vertical Scrollbar Visible"), "ColHdr"=w536) -> (error out=w539:errorcluster)  [unwired: 1 in, 1 out]
          }
          event "Tab Control": Value Change {
            w580 = TRUE ("Visible")
            w582 = FALSE ("Visible")
            w590 = TRUE ("Visible")
            w588 = FALSE ("Visible")
            n332 = event-data() -> ()  [unwired: 1 in, 5 out]
            n333 = property on="Select Names" class="Bool (strict)"(error in=w587, "Visible"=w588, "Value"=w588) -> (error out=w591:errorcluster)  [unwired: 1 in, 1 out]
            n334 = property on="Show Names" class="Bool (strict)"(error in=w591, "Visible"=w590) -> (error out=w589:errorcluster)  [unwired: 1 in, 1 out]
            n335 = property on="Experiment Name:" class="LstBox (strict)"(error in=w589, "ColHdrVis"=w590, "Height"=u32 25 ("Size:Height"), "Scrollbar Visible"=FALSE ("Visible Items:Vertical Scrollbar Visible")) -> (error out=w578:errorcluster)  [unwired: 1 in, 1 out]
            n336 = property on="Waveform Select Names" class="Bool (strict)"(error in=w578, "Visible"=w582, "Value"=w582) -> (error out=w579:errorcluster)  [unwired: 1 in, 1 out]
            n337 = property on="Waveform Show Names" class="Bool (strict)"(error in=w579, "Visible"=w580) -> (error out=w581:errorcluster)  [unwired: 1 in, 1 out]
            n338 = property on="Experiment Name:" class="LstBox (strict)"(error in=w581, "ColHdrVis"=w580, "Height"=u32 25 ("Size:Height"), "Scrollbar Visible"=FALSE ("Visible Items:Vertical Scrollbar Visible")) -> (error out=w577:errorcluster)  [unwired: 1 in, 1 out]
          }
          event "Small?", "If this was the big acc...": Value Change {
            # "Disable all waveforms-related elements\nunless this computer has access to big acc\ndata and is on the big acc, or this computer\nhas access to small data and is on the small acc."
            n339 = event-data() -> ()  [unwired: 1 in, 6 out]
            n340 = property on="Updating..." class="Bool (strict)"(error in=w616, "Value"=TRUE ("Updating...")) -> (error out=w609:errorcluster)  [unwired: 1 in, 1 out]
            n341 = String To IP(1:"" ("name")) -> (0:w604:u32)
            n342 = IP To String(2:w604) -> (0:w602:string)  [unwired: 1 in]
            n343 = Not(x="If this was the big acc...") -> (.not. x?=w612:bool)
            n344 = Equal?(x="NPL-PC-2", y=w602) -> (x = y?=w600:bool)
            n345 = And(x=w612, y="Small?") -> (x .and. y?=w611:bool)
            n346 = case shown="True" w611 {
              tunnel: [w629 w636] -> w608
              tunnel: w609 -> [w634 w641]
              frame True {
                n347 = property on="Constrained Distribution" class="XYGraph (strict)"(error in=w634, "XScale.Minimum"=0.001 ("X Scale.Range:Minimum"), "XScale.Maximum"=100.0 ("X Scale.Range:Maximum")) -> (error out=w628:errorcluster)  [unwired: 1 in, 1 out]
                n348 = property on="Pelletron Voltage (MV):" class="DigNum (strict)"(error in=w628, "Value"=0.005 ("Pelletron Voltage (MV):"), "Caption.Text"="Needle Voltage (MV):") -> (error out=w629:errorcluster)  [unwired: 1 in, 1 out]
              }
              frame False {
                n349 = property on="Constrained Distribution" class="XYGraph (strict)"(error in=w641, "XScale.Minimum"=0.1 ("X Scale.Range:Minimum"), "XScale.Maximum"=200.0 ("X Scale.Range:Maximum")) -> (error out=w635:errorcluster)  [unwired: 1 in, 1 out]
                n350 = property on="Pelletron Voltage (MV):" class="DigNum (strict)"(error in=w635, "Value"=2.17 ("Pelletron Voltage (MV):"), "Caption.Text"="Pelletron Voltage (MV):") -> (error out=w636:errorcluster)  [unwired: 1 in, 1 out]
              }
            }
            n351 = Equal?(x="Small?", y=w600) -> (x = y?=w598:bool)
            n352 = Select(t=T5."Enabled" ("Disabled"), s=w598, f=T5."Disabled and Grayed Out") -> (s? t:f=w595:T5)
            n353 = property on="Waveforms" class="Arr (strict)"("DisabledEnum"=w595) -> ()  [unwired: 2 in, 2 out]
            n354 = property on="Waveform Constraints" class="Clust (strict)"("DisabledEnum"=w595) -> ()  [unwired: 2 in, 2 out]
            n355 = property on="Plot Waveforms" class="Bool (strict)"("DisabledEnum"=w595) -> ()  [unwired: 2 in, 2 out]
            n356 = case shown="False" "Small?" {
              tunnel: w608 -> [w624 w626]
              tunnel: [w623 w625] -> w607
              frame False {
                w622 = FALSE ("If this was the big acc...")
                n357 = property on="If this was the big acc..." class="Bool (strict)"(error in=w624, "Value"=w622, "Visible"=w622) -> (error out=w623:errorcluster)  [unwired: 1 in, 1 out]
              }
              frame True {
                n358 = property on="If this was the big acc..." class="Bool (strict)"(error in=w626, "Visible"=TRUE) -> (error out=w625:errorcluster)  [unwired: 1 in, 1 out]
              }
            }
            n359 = property on="Waveform Show Names" class="Bool (strict)"("DisabledEnum"=w595) -> ()  [unwired: 2 in, 2 out]
            n360 = property on="Waveforms Experiment Group" class="Str"("DisabledEnum"=w595) -> ()  [unwired: 2 in, 2 out]
            n361 = property on="Waveforms Experiment Name" class="Str"("DisabledEnum"=w595) -> ()  [unwired: 2 in, 2 out]
            n362 = property on="Waveform Select Names" class="Bool (strict)"("DisabledEnum"=w595) -> ()  [unwired: 2 in, 2 out]
            n363 = property on="Select None" class="Bool"("DisabledEnum"=w595) -> ()  [unwired: 2 in, 2 out]
            n364 = property on="Limit waveforms to" class="DigNum (strict)"("DisabledEnum"=w595) -> ()  [unwired: 2 in, 2 out]
            n365 = property on="Selected?" class="Bool (strict)"("DisabledEnum"=w595) -> ()  [unwired: 2 in, 2 out]
            n366 = property on="Select All" class="Bool"("DisabledEnum"=w595) -> ()  [unwired: 2 in, 2 out]
            n367 = property on="Tab Control" class="TabCtl (strict)"(error in=w607, "Value"=T1."Query and Plot" ("Tab Control")) -> (error out=w614:errorcluster)  [unwired: 1 in, 1 out]
            n368 = property on="Set to plot constraints" class="Bool (strict)"("DisabledEnum"=w595) -> ()  [unwired: 2 in, 2 out]
            n369 = call-poly <userlib>:"Data Changed__ogtk.vi"("Boolean"="Small?") -> ("Changed"=w606:bool)
            n370 = case shown="True" w606 {
              tunnel: w614 -> [w618 w620]
              tunnel: [w618 w619] -> w613
              frame False {
              }
              frame True {
                n371 = property on="Reset Constraints to Default" class="Bool (strict)"(error in=w620, "Val(Sgnl)"=TRUE ("Updating...")) -> (error out=w619:errorcluster)  [unwired: 1 in, 1 out]
              }
            }
            n372 = property on="Show errored waveforms" class="Bool (strict)"("DisabledEnum"=w595) -> ()  [unwired: 2 in, 2 out]
            n373 = property on="Save Plot Waveforms" class="Bool (strict)"("DisabledEnum"=w595) -> ()  [unwired: 2 in, 2 out]
            n374 = property on="Save Selected Waveforms" class="Bool (strict)"("DisabledEnum"=w595) -> ()  [unwired: 2 in, 2 out]
            n375 = property on="Save Selected Metadata" class="Bool (strict)"("DisabledEnum"=w595) -> ()  [unwired: 2 in, 2 out]
            n376 = property on="Plot" class="Bool (strict)"(error in=w613, "Val(Sgnl)"=TRUE ("Updating...")) -> (error out=w592:errorcluster)  [unwired: 1 in, 1 out]
            n377 = property on="Plot Waveforms" class="Bool (strict)"(error in=w592, "Val(Sgnl)"=TRUE ("Updating...")) -> (error out=w593:errorcluster)  [unwired: 1 in, 1 out]
          }
          event Cursor Grab; Cursor Move {
            n378 = event-data() -> ()  [unwired: 1 in, 9 out]
            n379 = property on="Constrained Distribution" class="XYGraph (strict)"(error in=w647) -> (error out=w652:errorcluster, "Cursor.Cursor Y"=w651:dbl, "Cursor.Cursor X"=w650:dbl)  [unwired: 1 in, 1 out]
            n380 = local read "Density (g/cc)"() -> (w642:dbl)
            n381 = local read "Dust Type"() -> (w648:string)
            n382 = local write "Velocity (km/s)"(w650) -> ()
            n383 = local write "Mass (kg)"(w651) -> ()
            n384 = Not Equal To 0?(x=w642) -> (x != 0?=w645:bool)
            n385 = Equal?(x=w648, y="Multiple Dust Type" ("t")) -> (x = y?=w643:bool)
            n386 = And(x=w643, y=w645) -> (x .and. y?=w644:bool)
            n387 = case shown="False" w644 {
              tunnel: [w654 w689] -> w646
              tunnel: w652 -> [w653 w688]
              frame False {
                n388 = property on="Constrained Distribution" class="XYGraph (strict)"(error in=w653, "ActYScl"=0 ("Active Y Scale")) -> (error out=w679:errorcluster)  [unwired: 1 in, 1 out]
                n389 = local read "Density (g/cc)"() -> (w659:dbl)
                n390 = property on="Constrained Distribution" class="XYGraph (strict)"(error in=w679) -> (error out=w677:errorcluster, "YScale.Maximum"=w672:dbl, "YScale.Minimum"=w671:dbl, "Cursor.Cursor Y"=w660:dbl)  [unwired: 1 in, 1 out]
                n391 = Multiply(x=w659, y=1000.0) -> (x*y=w658:dbl)
                n392 = Build Array(w672, w671, w660) -> (w670:dbl[])
                n393 = Multiply(x=w670, y=3.0) -> (x*y=w686:dbl[])
                n394 = Divide(x=w686, y=4.0) -> (x/y=w665:dbl[])
                n395 = property on="Constrained Distribution" class="XYGraph (strict)"(error in=w677, "ActYScl"=1 ("Active Y Scale")) -> (error out=w676:errorcluster)  [unwired: 1 in, 1 out]
                n396 = Divide(x=w665, y=w658) -> (x/y=w685:dbl[])
                n397 = Divide(x=w685, y=3.141592653589793) -> (x/y=w683:dbl[])
                n398 = Y-th Root of X(1:w683, 2:3.0 ("x")) -> (0:w682:dbl[])
                n399 = Multiply(x=w682, y=1000000.0) -> (x*y=w668:dbl[])
                n400 = Index Array(array=w668) -> (element #1=w669:dbl, element #2=w667:dbl, element #3=w661:dbl)  [unwired: 3 in]
                n401 = property on="Constrained Distribution" class="XYGraph (strict)"(error in=w676, "YScale.Maximum"=w669, "YScale.Minimum"=w667, "YScale.Visible"=TRUE ("Y Scale.Visible")) -> (error out=w662:errorcluster)  [unwired: 1 in, 1 out]
                n402 = property on="Constrained Distribution" class="XYGraph (strict)"(error in=w662, "ActYScl"=0 ("Active Y Scale")) -> (error out=w673:errorcluster)  [unwired: 1 in, 1 out]
                n403 = property on="Radius (µm)" class="DigNum (strict)"(error in=w673, "DisabledEnum"=T5."Enabled" ("Disabled"), "Value"=w661) -> (error out=w655:errorcluster)  [unwired: 1 in, 1 out]
                n404 = property on="Density (g/cc)" class="DigNum (strict)"(error in=w655, "Visible"=TRUE) -> (error out=w654:errorcluster)  [unwired: 1 in, 1 out]
              }
              frame True {
                n405 = property on="Constrained Distribution" class="XYGraph (strict)"(error in=w688, "ActYScl"=1 ("Active Y Scale")) -> (error out=w696:errorcluster)  [unwired: 1 in, 1 out]
                n406 = property on="Constrained Distribution" class="XYGraph (strict)"(error in=w696, "YScale.Visible"=FALSE ("Y Scale.Visible")) -> (error out=w694:errorcluster)  [unwired: 1 in, 1 out]
                n407 = property on="Constrained Distribution" class="XYGraph (strict)"(error in=w694, "ActYScl"=0 ("Active Y Scale")) -> (error out=w691:errorcluster)  [unwired: 1 in, 1 out]
                n408 = property on="Radius (µm)" class="DigNum (strict)"(error in=w691, "DisabledEnum"=T5."Disabled and Grayed Out" ("Disabled")) -> (error out=w690:errorcluster)  [unwired: 1 in, 1 out]
                n409 = property on="Density (g/cc)" class="DigNum (strict)"(error in=w690, "Visible"=FALSE) -> (error out=w689:errorcluster)  [unwired: 1 in, 1 out]
              }
            }
          }
          event "Mass (kg)", "Velocity (km/s)": Value Change {
            n410 = event-data() -> ()  [unwired: 1 in, 5 out]
            n411 = local read "Density (g/cc)"() -> (w708:dbl)
            n412 = property on="Constrained Distribution" class="XYGraph (strict)"(error in=w700, "Cursor.Cursor X"="Velocity (km/s)", "Cursor.Cursor Y"="Mass (kg)") -> (error out=w699:errorcluster)  [unwired: 1 in, 1 out]
            n413 = Multiply(x=w708, y=1000.0) -> (x*y=w707:dbl)
            n414 = Multiply(x="Mass (kg)", y=3.0) -> (x*y=w701:dbl)
            n415 = Divide(x=w701, y=4.0) -> (x/y=w709:dbl)
            n416 = Divide(x=w709, y=w707) -> (x/y=w715:dbl)
            n417 = Divide(x=w715, y=3.141592653589793) -> (x/y=w713:dbl)
            n418 = Y-th Root of X(1:w713, 2:3.0 ("y")) -> (0:w712:dbl)
            n419 = Multiply(x=w712, y=1000000.0) -> (x*y=w704:dbl)
            n420 = local write "Radius (µm)"(w704) -> ()
          }
          event "Radius (µm)": Value Change {
            n421 = event-data() -> ()  [unwired: 1 in, 5 out]
            n422 = local read "Density (g/cc)"() -> (w722:dbl)
            n423 = Divide(x="Radius (µm)", y=1000000.0) -> (x/y=w725:dbl)
            n424 = Power Of X(1:w725, 2:3.0 ("y")) -> (0:w724:dbl)
            n425 = Multiply(x=w724, y=4.0) -> (x*y=w732:dbl)
            n426 = Multiply(x=1000.0, y=w722) -> (x*y=w720:dbl)
            n427 = Divide(x=w732, y=3.0) -> (x/y=w730:dbl)
            n428 = Multiply(x=w730, y=3.141592653589793) -> (x*y=w723:dbl)
            n429 = Multiply(x=w723, y=w720) -> (x*y=w718:dbl)
            n430 = property on="Constrained Distribution" class="XYGraph (strict)"(error in=w717, "Cursor.Cursor Y"=w718) -> (error out=w721:errorcluster)  [unwired: 1 in, 1 out]
            n431 = local write "Mass (kg)"(w718) -> ()
          }
          event "Limit no. of\nplotted events": Value Change {
            n432 = event-data() -> ()  [unwired: 1 in, 6 out]
            n433 = Select(t=T5."Enabled" ("Disabled"), s="Limit no. of\nplotted events", f=T5."Disabled and Grayed Out" ("Disabled")) -> (s? t:f=w735:T5)
            n434 = property on="Limit to" class="DigNum (strict)"(error in=w739, "DisabledEnum"=w735) -> (error out=w734:errorcluster)  [unwired: 1 in, 1 out]
          }
          event "Save Plot Waveforms": Value Change {
            n435 = event-data() -> ()  [unwired: 1 in, 5 out]
            n436 = local read "Limit no. of\nplotted events"() -> (w756:bool)
            n437 = local read "Constraints"() -> (w754:T3)
            n438 = local read "Small?"() -> (w753:bool)
            n439 = local read "Limit to"() -> (w750:i64)
            n440 = property on="Updating..." class="Bool (strict)"(error in=w761, "Value"=TRUE ("Updating...")) -> (error out=w757:errorcluster)  [unwired: 1 in, 1 out]
            n441 = call "Count_Events.vi"("Small?"=w753, "Constraints"=w754) -> ("Number of Events"=w751:u64)  [unwired: 8 in, 1 out]
            n442 = Less?(x=w750, y=w751) -> (x < y?=w749:bool)
            n443 = And(x=w756, y=w749) -> (x .and. y?=w752:bool)
            n444 = case shown="True" w752 {
              tunnel: [w763 w770] -> w748
              tunnel: w757 -> [w763 w770]
              tunnel: [FALSE ("T button?") w769] -> w755
              frame False {
              }
              frame True {
                n445 = local read "Limit to"() -> (w766:i64)
                n446 = Format Into String(format string="Limit to %d events?" ("message"), w766) -> (resulting string=w768:string)  [unwired: 2 in, 1 out]
                n447 = Two Button Dialog(message=w768, 1:"No" ("F button name (\"Cancel\")"), 2:"Yes" ("T button name (\"OK\")")) -> (T button?=w769:bool)
              }
            }
            n448 = call "Save_File_Dialog.vi"("error in (no error)"=w748, "Filename"="New_Database_Query.hdf5") -> ("error out"=w747:errorcluster, "Cancelled"=w746:bool, "Path"=w745:path)  [unwired: 7 in]
            n449 = case shown="False" w746 {
              tunnel: [w774 w806] -> w759
              tunnel: w747 -> [w777 w806]
              tunnel: w745 -> [w782 _]
              tunnel: w755 -> [w786 _]
              frame False {
                n450 = property on="Save Plot Waveforms" class="Bool (strict)"(error in=w777, "BoolText.Text"="Searching..." ("Boolean Text.Text")) -> (error out=w776:errorcluster)  [unwired: 1 in, 1 out]
                n451 = local read "Constraints"() -> (w788:T3)
                n452 = local read "Limit to"() -> (w785:i64)
                n453 = local read "Small?"() -> (w787:bool)
                n454 = call "dust_event_query.vi"("No. of Events"=w785, "error in (no error)"=w776, "Limited?"=w786, "Small?"=w787, "Constraints"=w788) -> ("error out"=w783:errorcluster, "Dust Event ID Array"=w778:i64[], "Dust Array"=w771:T8[])  [unwired: 2 in, 2 out]
                n455 = call <vilib>:"H5F_open.vi"("error in (no error)"=w783, "mode"=H5F_mode."overwrite", "path"=w782) -> ("error out"=w772:errorcluster, "ref"=w784:i32)  [unwired: 1 in]
                n456 = for {
                  N -> [w796]
                  tunnel: w778 -> [w793] mode=indexing
                  shift-right: [w795] -> w773
                  shift-left: w772 -> [w794]
                  shift-right: [w791] -> w780
                  shift-left: w784 -> [w792]
                  tunnel: w771 -> [w789] mode=indexing
                  i -> [w797]
                  n457 = call "Save_Waveforms.vi"("Cluster"=w789, "error in (no error)"=w794, "id_dust_event"=w793, "ref"=w792) -> ("error out"=w790:errorcluster, "ref out"=w791:i32)  [unwired: 6 in]
                  n458 = Increment(x=w797) -> (x+1=w801:i32)
                  n459 = Divide(x=w801, y=w796) -> (x/y=w799:dbl)
                  n460 = Multiply(x=w799, y=100) -> (x*y=w805:dbl)
                  "Plotted Waveforms Slide" <- w805
                  n461 = Number To Decimal String(number=w805) -> (decimal integer string=w802:string)  [unwired: 1 in]
                  n462 = Concatenate Strings("Writing...\n" ("string"), w802, "% Complete." ("string")) -> (w798:string)
                  n463 = property on="Save Plot Waveforms" class="Bool (strict)"(error in=w790, "BoolText.Text"=w798) -> (error out=w795:errorcluster)  [unwired: 1 in, 1 out]
                }
                n464 = call <vilib>:"H5F_close.vi"("error in (no error)"=w772, "ref"=w780) -> ("error out"=w779:errorcluster)  [unwired: 3 in]
                n465 = Merge Errors(w773, w779) -> (w774:errorcluster)
              }
              frame True {
              }
            }
            n466 = property on="Save Plot Waveforms" class="Bool (strict)"(error in=w759, "BoolText.Text"="Save Waveforms" ("f"), "Value"=FALSE ("Save Plotted Waveforms")) -> (error out=w758:errorcluster)  [unwired: 1 in, 1 out]
            n467 = property on="Plotted Waveforms Slide" class="Slide (strict)"(error in=w758, "Value"=u8 0 ("Waveforms Slide")) -> (error out=w741:errorcluster)  [unwired: 1 in, 1 out]
          }
          event "Save Plot Metadata": Value Change {
            n468 = event-data() -> ()  [unwired: 1 in, 5 out]
            n469 = local read "Constraints"() -> (w820:T3)
            n470 = local read "Limit no. of\nplotted events"() -> (w824:bool)
            n471 = local read "Small?"() -> (w816:bool)
            n472 = local read "Limit to"() -> (w818:i64)
            n473 = property on="Updating..." class="Bool (strict)"(error in=w825, "Value"=TRUE ("Updating...")) -> (error out=w823:errorcluster)  [unwired: 1 in, 1 out]
            n474 = call "Count_Events.vi"("Small?"=w816, "Constraints"=w820) -> ("Number of Events"=w819:u64)  [unwired: 8 in, 1 out]
            n475 = Less?(x=w818, y=w819) -> (x < y?=w817:bool)
            n476 = And(x=w824, y=w817) -> (x .and. y?=w821:bool)
            n477 = case shown="True" w821 {
              tunnel: [FALSE ("T button?") w838] -> w822
              tunnel: [w830 w834] -> w815
              tunnel: w823 -> [w830 w834]
              frame False {
              }
              frame True {
                n478 = local read "Limit to"() -> (w835:i64)
                n479 = Format Into String(format string="Limit to %d events?" ("message"), w835) -> (resulting string=w837:string)  [unwired: 2 in, 1 out]
                n480 = Two Button Dialog(message=w837, 1:"No" ("F button name (\"Cancel\")"), 2:"Yes" ("T button name (\"OK\")")) -> (T button?=w838:bool)
              }
            }
            n481 = local read "Last Metadata Name"() -> (w814:string)
            n482 = call "Save_File_Dialog.vi"("error in (no error)"=w815, "Filename"=w814) -> ("error out"=w811:errorcluster, "Cancelled"=w812:bool, "Path"=w813:path)  [unwired: 7 in]
            n483 = Strip Path(path=w813) -> (name=→"Last Metadata Name":string)  [unwired: 1 out]
            n484 = case shown="False" w812 {
              tunnel: w813 -> [w850 _]
              tunnel: w811 -> [w841 w868]
              tunnel: [w848 w868] -> w828
              tunnel: w822 -> [w844 _]
              frame False {
                n485 = local read "Constraints"() -> (w846:T3)
                n486 = local read "Small?"() -> (w842:bool)
                n487 = local read "Limit to"() -> (w843:i64)
                n488 = call "make_metadata_array.vi"() -> ("Header Array"=w840:string[])  [unwired: 3 in, 1 out]
                n489 = call-poly <vilib>:"Write To Spreadsheet File.vi"("delimiter (\\t)"="," ("delimiter (\\t)"), "1D data"=w840, "file path (dialog if empty)"=w850) -> ("new file path (Not A Path if cancelled)"=w839:path)  [unwired: 5 in]
                n490 = call "dust_event_query.vi"("No. of Events"=w843, "error in (no error)"=w841, "Limited?"=w844, "Small?"=w842, "Constraints"=w846) -> ("error out"=w849:errorcluster, "Dust Array"=w845:T8[])  [unwired: 2 in, 3 out]
                n491 = for {
                  N -> [w856]
                  tunnel: w845 -> [w855] mode=indexing
                  shift-right: [w861] -> w848
                  shift-left: w849 -> [w857]
                  tunnel: w839 -> [w853]
                  i -> [w859]
                  n492 = call "make_metadata_array.vi"("Cluster"=w855) -> ("Metadata Array"=w852:string[])  [unwired: 2 in, 1 out]
                  n493 = Increment(x=w859) -> (x+1=w858:i32)
                  n494 = call-poly <vilib>:"Write To Spreadsheet File.vi"("delimiter (\\t)"="," ("delimiter (\\t)"), "append to file? (new file:F)"=TRUE, "1D data"=w852, "file path (dialog if empty)"=w853) -> ()  [unwired: 4 in, 1 out]
                  n495 = Divide(x=w858, y=w856) -> (x/y=w862:dbl)
                  n496 = Multiply(x=w862, y=100) -> (x*y=w860:dbl)
                  "Plotted Metadata Slide" <- w860
                  n497 = Number To Decimal String(number=w860) -> (decimal integer string=w864:string)  [unwired: 1 in]
                  n498 = Concatenate Strings("Writing...\n" ("string"), w864, "% Complete." ("string")) -> (w867:string)
                  n499 = property on="Save Plot Metadata" class="Bool (strict)"(error in=w857, "BoolText.Text"=w867) -> (error out=w861:errorcluster)  [unwired: 1 in, 1 out]
                }
              }
              frame True {
              }
            }
            n500 = property on="Save Plot Metadata" class="Bool (strict)"(error in=w828, "BoolText.Text"="Save Metadata" ("Boolean Text.Text"), "Value"=FALSE ("Save Plot Metadata")) -> (error out=w808:errorcluster)  [unwired: 1 in, 1 out]
            n501 = property on="Plotted Metadata Slide" class="Slide (strict)"(error in=w808, "Value"=u8 0 ("Waveforms Slide")) -> (error out=w807:errorcluster)  [unwired: 1 in, 1 out]
          }
          event "Save Image": Value Change {
            n502 = event-data() -> ()  [unwired: 1 in, 5 out]
            n503 = property on="Updating..." class="Bool (strict)"(error in=w877, "Value"=TRUE ("Updating...")) -> (error out=w876:errorcluster)  [unwired: 1 in, 1 out]
            n504 = invoke on="Constrained Distribution" class="XYGraph (strict)" method="Get Image"(error in=w876) -> (error out=w875:errorcluster, "image data"=w880:T12)  [unwired: 5 in, 4 out]
            n505 = call "Save_File_Dialog.vi"("error in (no error)"=w875, "Filename"="Distribution.png") -> ("error out"=w873:errorcluster, "Cancelled"=w871:bool, "Path"=w872:path)  [unwired: 7 in]
            n506 = case shown="False" w871 {
              tunnel: w880 -> [w884 _]
              tunnel: [w883 w885] -> w879
              tunnel: w873 -> [w882 w885]
              tunnel: w872 -> [w881 _]
              frame False {
                n507 = call <vilib>:"Write PNG File.vi"("error in (no error)"=w882, "image data"=w884, "path to PNG file"=w881) -> ("error out"=w883:errorcluster)  [unwired: 7 in, 1 out]
              }
              frame True {
              }
            }
            n508 = property on="Save Image" class="Bool (strict)"(error in=w879, "Value"=FALSE ("Save Image")) -> (error out=w870:errorcluster)  [unwired: 1 in, 1 out]
          }
          event "Waveforms": Key Down; "Waveforms": Mouse Down; "Waveforms": Mouse Up; "Waveforms": Key Up {
            # "This event is for when the user selects a different graph."
            # "Forces the y-scale of the graph\nto autoscale to the data."
            n509 = event-data() -> ()  [unwired: 1 in, 5 out]
            n510 = local read "Limit waveforms to"() -> (w893:i64)
            n511 = property on="Waveforms" class="Arr (strict)"(error in=w898) -> (error out=w888:errorcluster, "Value"=w887:T4[], "Index Values"=w895:u32[])  [unwired: 1 in, 1 out]
            n512 = call-poly <userlib>:"Empty Array__ogtk.vi"("Array"=w887) -> ("Empty Array?"=w894:bool)  [unwired: 8 in]
            n513 = case shown="False" w894 {
              tunnel: w895 -> [w914 _]
              tunnel: w893 -> [w905 _]
              tunnel: w888 -> [w908 w915]
              tunnel: w887 -> [w907 _]
              tunnel: [w904 w915] -> w886
              frame False {
                n514 = Index Array(array=w914) -> (element=w912:u32)  [unwired: 1 in]
                n515 = Decrement(x=w905) -> (x-1=w911:i64)
                n516 = Less?(x=w912, y=w911) -> (x < y?=w913:bool)
                n517 = Array Subset(array=w907, length=w905) -> (w906:T4[])  [unwired: 1 in]
                n518 = Select(t=w912, s=w913, f=w911) -> (s? t:f=w909:i64)
                n519 = Build Array(w909) -> (w910:i64[])
                n520 = property on="Waveforms" class="Arr (strict)"(error in=w908, "Value"=w906, "Index Values"=w910) -> (error out=w904:errorcluster)  [unwired: 1 in, 1 out]
              }
              frame True {
              }
            }
            n521 = property on="id_dust_event" class="DigNum (strict)"(error in=w886) -> (error out=w896:errorcluster, "Value"=w897:u64)  [unwired: 1 in, 1 out]
            n522 = property on="Selected Waveforms" class="Arr (strict)"(error in=w896) -> (error out=w902:errorcluster, "Value"=w903:u64[])  [unwired: 1 in, 1 out]
            n523 = call-poly <userlib>:"Search Array__ogtk.vi"("Array"=w903, "Element Data"=w897) -> ("Indices of Elements"=w901:i32[])  [unwired: 7 in]
            n524 = call-poly <userlib>:"Empty Array__ogtk.vi"("Array"=w901) -> ("Empty Array?"=w900:bool)  [unwired: 8 in]
            n525 = Not(x=w900) -> (.not. x?=w899:bool)
            n526 = property on="Selected?" class="Bool (strict)"(error in=w902, "Value"=w899) -> (error out=w892:errorcluster)  [unwired: 1 in, 1 out]
            n527 = property on="Waveform Graph" class="WFGraph (strict)"(error in=w892) -> (error out=w890:errorcluster, "Value"=w891:sgl[][])  [unwired: 1 in, 1 out]
            n528 = property on="Waveform Graph" class="WFGraph (strict)"(error in=w890, "Val(Sgnl)"=w891) -> (error out=w889:errorcluster)  [unwired: 1 in, 1 out]
          }
          event "Reset Visible Time": Value Change {
            n529 = event-data() -> ()  [unwired: 1 in, 6 out]
            n530 = local read "Max Time"() -> (w916:dbl)
            n531 = property on="Time Visible" class="DigNum (strict)"(error in=w917, "Val(Sgnl)"=w916) -> (error out=w918:errorcluster)  [unwired: 1 in, 1 out]
          }
          event "Time Visible": Value Change {
            n532 = event-data() -> ()  [unwired: 1 in, 6 out]
            n533 = property on="Waveform Graph" class="WFGraph (strict)"(error in=w926) -> (error out=w924:errorcluster, "XScale.Minimum"=w925:dbl)  [unwired: 1 in, 1 out]
            n534 = local read "Max Time"() -> (w919:dbl)
            n535 = Add(x=w925, y="Time Visible") -> (x+y=w920:dbl)
            n536 = Less Or Equal?(x=w920, y=w919) -> (x <= y?=w922:bool)
            n537 = case shown="False" w922 {
              tunnel: w920 -> [_ w934]
              tunnel: w924 -> [w932 w935]
              tunnel: [w931 w933] -> w923
              tunnel: "Time Visible" -> [w928 _]
              tunnel: w919 -> [w929 _]
              frame False {
                n538 = property on="Waveform Graph" class="WFGraph (strict)"(error in=w932, "XScale.Maximum"=w929) -> (error out=w930:errorcluster)  [unwired: 1 in, 1 out]
                n539 = Subtract(x=w929, y=w928) -> (x-y=w927:dbl)
                n540 = property on="Waveform Graph" class="WFGraph (strict)"(error in=w930, "XScale.Minimum"=w927) -> (error out=w931:errorcluster)  [unwired: 1 in, 1 out]
              }
              frame True {
                n541 = property on="Waveform Graph" class="WFGraph (strict)"(error in=w935, "XScale.Maximum"=w934) -> (error out=w933:errorcluster)  [unwired: 1 in, 1 out]
              }
            }
          }
          event "Selected?": Value Change {
            n542 = event-data() -> ()  [unwired: 1 in, 6 out]
            n543 = property on="Waveforms" class="Arr (strict)"(error in=w949) -> (error out=w948:errorcluster, "Value"=w946:T4[], "Index Values"=w945:u32[])  [unwired: 1 in, 1 out]
            n544 = Index Array(array=w945) -> (element=w944:u32)  [unwired: 1 in]
            n545 = Index Array(array=w946, index=w944) -> (element=w943:T4)
            n546 = Unbundle By Name(w943) -> ("id_dust_event"=w941:u64)
            n547 = property on="Selected Waveforms" class="Arr (strict)"(error in=w948) -> (error out=w947:errorcluster, "Value"=w942:u64[])  [unwired: 1 in, 1 out]
            n548 = call-poly <userlib>:"Search Array__ogtk.vi"("Array"=w942, "Element Data"=w941) -> ("Indices of Elements"=w940:i32[])  [unwired: 7 in]
            n549 = case shown="True" "Selected?" {
              tunnel: [w951 w957] -> w939
              tunnel: w947 -> [w951 w957]
              tunnel: w942 -> [w955 w959]
              tunnel: w941 -> [w952 _]
              tunnel: w940 -> [_ w958]
              tunnel: [w950 w956] -> w937
              frame True {
                n550 = Insert Into Array(array=w955, new element=w952) -> (w954:u64[])  [unwired: 1 in]
                n551 = call-poly <userlib>:"Sort Array__ogtk.vi"("Order"=enum16{"ascending", "descending"}."descending", "Array in"=w954) -> ("Sorted Array out"=w950:u64[])  [unwired: 8 in, 1 out]
              }
              frame False {
                n552 = call-poly <userlib>:"Delete Elements from Array__ogtk.vi"("indices"=w958, "array"=w959) -> ("array w/ subset deleted"=w956:u64[])  [unwired: 8 in, 1 out]
              }
            }
            n553 = property on="Selected Waveforms" class="Arr (strict)"(error in=w939, "Val(Sgnl)"=w937) -> (error out=w938:errorcluster)  [unwired: 1 in, 1 out]
          }
          event "Select All": Value Change {
            n554 = event-data() -> ()  [unwired: 1 in, 6 out]
            n555 = property on="Waveforms" class="Arr (strict)"(error in=w967) -> (error out=w965:errorcluster, "Value"=w966:T4[])  [unwired: 1 in, 1 out]
            n556 = for {
              tunnel: w966 -> [w970] mode=indexing
              shift-right: [w969] -> w964
              shift-left: w965 -> [w969]
              tunnel: [w968] -> w963 mode=indexing
              n557 = Unbundle By Name(w970) -> ("id_dust_event"=w968:u64)
            }
            n558 = property on="Selected Waveforms" class="Arr (strict)"(error in=w964, "Val(Sgnl)"=w963) -> (error out=w962:errorcluster)  [unwired: 1 in, 1 out]
            n559 = property on="Selected?" class="Bool (strict)"(error in=w962, "Value"=TRUE ("Selected?")) -> (error out=w960:errorcluster)  [unwired: 1 in, 1 out]
          }
          event "Select None": Value Change {
            n560 = event-data() -> ()  [unwired: 1 in, 6 out]
            n561 = property on="Selected Waveforms" class="Arr (strict)"(error in=w974, "Val(Sgnl)"=u64[] [] ("Value (Signaling)")) -> (error out=w972:errorcluster)  [unwired: 1 in, 1 out]
            n562 = property on="Selected?" class="Bool (strict)"(error in=w972, "Value"=FALSE ("Selected?")) -> (error out=w971:errorcluster)  [unwired: 1 in, 1 out]
          }
          event "Selected Waveforms": Value Change {
            n563 = event-data() -> ()  [unwired: 1 in, 6 out]
            n564 = property on="Plot" class="Bool (strict)"(error in=w980, "Val(Sgnl)"=TRUE ("Value (Signaling)")) -> (error out=w979:errorcluster)  [unwired: 1 in, 1 out]
            n565 = property on="Selected Waveforms" class="Arr (strict)"(error in=w979) -> (error out=w976:errorcluster, "Value"=w977:u64[])  [unwired: 1 in, 1 out]
            n566 = Array Size(array=w977) -> (size(s)=→"Number of selected waveforms":i32)
          }
          event "Save Selected Waveforms": Value Change {
            n567 = event-data() -> ()  [unwired: 1 in, 6 out]
            n568 = property on="Updating..." class="Bool (strict)"(error in=w983, "Value"=TRUE ("Updating...")) -> (error out=w982:errorcluster)  [unwired: 1 in, 1 out]
            n569 = call "Save_File_Dialog.vi"("error in (no error)"=w982, "Filename"="New_Database_Query.hdf5") -> ("error out"=w992:errorcluster, "Cancelled"=w991:bool, "Path"=w990:path)  [unwired: 7 in]
            n570 = case shown="False" w991 {
              tunnel: [w1000 w1026] -> w993
              tunnel: w992 -> [w1003 w1026]
              tunnel: w990 -> [w1007 _]
              frame False {
                n571 = local read "Selected Waveforms"() -> (w997:u64[])
                n572 = local read "Small?"() -> (w995:bool)
                n573 = property on="Save Selected Waveforms" class="Bool (strict)"(error in=w1003, "BoolText.Text"="Searching..." ("Boolean Text.Text")) -> (error out=w1001:errorcluster)  [unwired: 1 in, 1 out]
                n574 = call <vilib>:"H5F_open.vi"("error in (no error)"=w1001, "mode"=H5F_mode."overwrite", "path"=w1007) -> ("error out"=w998:errorcluster, "ref"=w1008:i32)  [unwired: 1 in]
                n575 = call "selected_dust_events_query.vi"("Small?"=w995, "Dust Events"=w997) -> ("Dust Array"=w996:T8[])  [unwired: 5 in, 4 out]
                n576 = for {
                  N -> [w1017]
                  tunnel: w997 -> [w1015] mode=indexing
                  shift-right: [w1016] -> w999
                  shift-left: w998 -> [w1009]
                  shift-right: [w1013] -> w1005
                  shift-left: w1008 -> [w1014]
                  tunnel: w996 -> [w1010] mode=indexing
                  i -> [w1018]
                  n577 = call "Save_Waveforms.vi"("Cluster"=w1010, "error in (no error)"=w1009, "id_dust_event"=w1015, "ref"=w1014) -> ("error out"=w1012:errorcluster, "ref out"=w1013:i32)  [unwired: 6 in]
                  n578 = Increment(x=w1018) -> (x+1=w1022:i32)
                  n579 = Divide(x=w1022, y=w1017) -> (x/y=w1020:dbl)
                  n580 = Multiply(x=w1020, y=100) -> (x*y=w1011:dbl)
                  "Selected Waveforms Slide" <- w1011
                  n581 = Number To Decimal String(number=w1011) -> (decimal integer string=w1023:string)  [unwired: 1 in]
                  n582 = Concatenate Strings("Writing...\n" ("string"), w1023, "% Complete." ("string")) -> (w1019:string)
                  n583 = property on="Save Selected Waveforms" class="Bool (strict)"(error in=w1012, "BoolText.Text"=w1019) -> (error out=w1016:errorcluster)  [unwired: 1 in, 1 out]
                }
                n584 = call <vilib>:"H5F_close.vi"("error in (no error)"=w998, "ref"=w1005) -> ("error out"=w1004:errorcluster)  [unwired: 3 in]
                n585 = Merge Errors(w999, w1004) -> (w1000:errorcluster)
              }
              frame True {
              }
            }
            n586 = property on="Save Selected Waveforms" class="Bool (strict)"(error in=w993, "BoolText.Text"="Save Waveforms" ("f"), "Value"=FALSE ("Save Selected Waveforms")) -> (error out=w986:errorcluster)  [unwired: 1 in, 1 out]
            n587 = property on="Selected Waveforms Slide" class="Slide (strict)"(error in=w986, "Value"=u8 0 ("Waveforms Slide")) -> (error out=w985:errorcluster)  [unwired: 1 in, 1 out]
          }
          event "Save Selected Metadata": Value Change {
            n588 = event-data() -> ()  [unwired: 1 in, 6 out]
            n589 = local read "Last Metadata Name"() -> (w1038:string)
            n590 = property on="Updating..." class="Bool (strict)"(error in=w1027, "Value"=TRUE ("Updating...")) -> (error out=w1028:errorcluster)  [unwired: 1 in, 1 out]
            n591 = call "Save_File_Dialog.vi"("error in (no error)"=w1028, "Filename"=w1038) -> ("error out"=w1035:errorcluster, "Cancelled"=w1036:bool, "Path"=w1037:path)  [unwired: 7 in]
            n592 = case shown="False" w1036 {
              tunnel: w1037 -> [w1051 _]
              tunnel: w1035 -> [w1043 w1069]
              tunnel: [w1050 w1069] -> w1040
              frame False {
                n593 = local read "Selected Waveforms"() -> (w1046:u64[])
                n594 = property on="Save Selected Metadata" class="Bool (strict)"(error in=w1043, "BoolText.Text"="Searching..." ("Boolean Text.Text")) -> (error out=w1044:errorcluster)  [unwired: 1 in, 1 out]
                n595 = call "make_metadata_array.vi"() -> ("Header Array"=w1042:string[])  [unwired: 3 in, 1 out]
                n596 = call-poly <vilib>:"Write To Spreadsheet File.vi"("delimiter (\\t)"="," ("delimiter (\\t)"), "1D data"=w1042, "file path (dialog if empty)"=w1051) -> ("new file path (Not A Path if cancelled)"=w1041:path)  [unwired: 5 in]
                n597 = call "selected_dust_events_query.vi"("error in (no error)"=w1044, "Dust Events"=w1046) -> ("error out"=w1048:errorcluster, "Dust Array"=w1047:T8[])  [unwired: 5 in, 3 out]
                n598 = for {
                  N -> [w1058]
                  tunnel: w1047 -> [w1056] mode=indexing
                  shift-right: [w1062] -> w1050
                  shift-left: w1048 -> [w1059]
                  tunnel: w1041 -> [w1052]
                  i -> [w1061]
                  n599 = call "make_metadata_array.vi"("Cluster"=w1056) -> ("Metadata Array"=w1054:string[])  [unwired: 2 in, 1 out]
                  n600 = Increment(x=w1061) -> (x+1=w1060:i32)
                  n601 = Divide(x=w1060, y=w1058) -> (x/y=w1063:dbl)
                  n602 = call-poly <vilib>:"Write To Spreadsheet File.vi"("delimiter (\\t)"="," ("delimiter (\\t)"), "append to file? (new file:F)"=TRUE, "1D data"=w1054, "file path (dialog if empty)"=w1052) -> ()  [unwired: 4 in, 1 out]
                  n603 = Multiply(x=w1063, y=100) -> (x*y=w1057:dbl)
                  "Selected Metadata Slide" <- w1057
                  n604 = Number To Decimal String(number=w1057) -> (decimal integer string=w1065:string)  [unwired: 1 in]
                  n605 = Concatenate Strings("Writing...\n" ("string"), w1065, "% Complete." ("string")) -> (w1068:string)
                  n606 = property on="Save Selected Metadata" class="Bool (strict)"(error in=w1059, "BoolText.Text"=w1068) -> (error out=w1062:errorcluster)  [unwired: 1 in, 1 out]
                }
              }
              frame True {
              }
            }
            n607 = Strip Path(path=w1037) -> (name=w1034:string)  [unwired: 1 out]
            n608 = local write "Last Metadata Name"(w1034) -> ()
            n609 = property on="Save Selected Metadata" class="Bool (strict)"(error in=w1040, "BoolText.Text"="Save Metadata" ("Boolean Text.Text"), "Value"=FALSE ("Save Selected Metadata")) -> (error out=w1031:errorcluster)  [unwired: 1 in, 1 out]
            n610 = property on="Selected Metadata Slide" class="Slide (strict)"(error in=w1031, "Value"=u8 0 ("Waveforms Slide")) -> (error out=w1030:errorcluster)  [unwired: 1 in, 1 out]
          }
          event "Exit": Value Change {
            n611 = event-data() -> ()  [unwired: 1 in, 6 out]
          }
        }
        n612 = case shown="No Error" w108 {
          selector: w108 -> [w113 w117]
          tunnel: [w113 w118] -> w107
          tunnel: [w112 w117] -> w106
          frame No Error {
            n613 = case shown="False" "Clear Errors" {
              tunnel: w113 -> [_ w116]
              tunnel: [w115 w116] -> w112
              frame False {
                n614 = local read "error out"() -> (w115:errorcluster)
              }
              frame True {
                n615 = local write "error out"(w116) -> ()
              }
            }
          }
          frame Error {
            n616 = call <vilib>:"Clear Errors.vi"("error in (no error)"=w117) -> ("error out"=w118:errorcluster)  [unwired: 5 in, 1 out]
            n617 = local write "error out"(w117) -> ()
          }
        }
      }
      n618 = property on="Exit" class="Bool (strict)"(error in=w104, "Value"=FALSE ("Exit")) -> ()  [unwired: 1 in, 2 out]
    }
    frame Error {
    }
  }
  "error out" <- w1
  "Max Time" <- w4
